vi "Main.vi"() -> ()   [LabVIEW 2017]
uses:
  Controls/MHLData.ctl
  Controls/objectRefsMain.ctl
  <vilib>/Utility/miscctls.llb/LVPositionTypeDef.ctl
  <vilib>/Utility/error.llb/DialogType.ctl
  7da0cd4f-55e9-4c1f-8356-bed5fd081df9.vi
  20102e64-79ad-4bb2-912e-c55f23ce2fb7.vi
  581ba121-4117-45c7-b05f-45eec266b530.vi
  Support/Configuration/globalConstants.vi
  <vilib>/Utility/error.llb/Error Cluster From Error Code.vi
  <vilib>/ErrorRing/Error Ring.xnode
  Support/Configuration/Message Queues/Message Queue.lvlib
  Support/Configuration/User Events/User Event - Stop.lvlib
  user32.dll
panel:
  in  "Excel._Application":refnum<k7>
  out "IL RL Standards":T1
  out "Channel Select":bool[](array[boolean])
  out "Save File":refnum<file>
  out "Device ID":refnum<visa-resource-name>="GPIB0::17::INSTR" caption="VISA resource name"
  out "experiorLogo":picture
  out "statusMessage":string="Loading Experior IL-RL"
  out "Running":bool
  in  "New Test":bool
  in  "Engineering Mode":bool
  in  "abort":bool caption="Abort"
  in  "Remeasure":bool caption="Redo"
  in  "Method Selection":u16(ring) items=["Select IL Method", "---------------------", "Standard IL", "Substitution"]
  in  "Standard Selection":u16(ring) items=["Select Test Standard", "---------------------", "No Standard", "Custom Standard", "---------------------", "GR326-UPC-New ", "GR326-UPC-During/End", "GR326-APC-New ", "GR326-APC-During/End", "GR1435-Standard-New", "GR1435-Standard-During/End"]
  in  "Rereference":bool caption="Redo"
  in  "Sample ID":string caption="Sample Number"
  in  "Enable RL":bool
  in  "Enable IL":bool
  in  "Enable Switch":bool
  in  "Wavelength Enable":T2
  in  "Channel Cluster":T3
  in  "Save Data":bool
  in  "Take Measurement":bool
  in  "Take Reference":bool
  in  "menuSlider":bool
  in  "moduleSlider":bool
  in  "Open Save":bool
  out "Save Path":string="C:\\_Labtech\\"
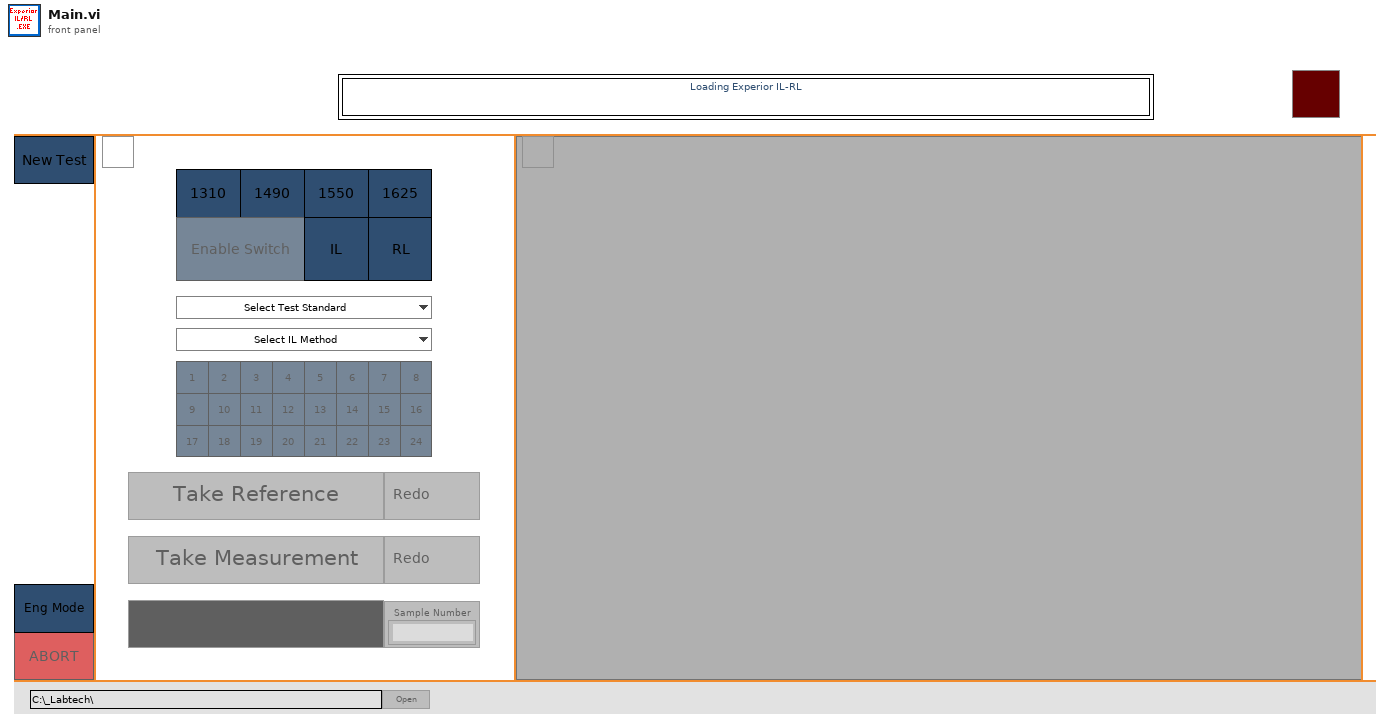
[diagram p1: front panel]
types:
  T1 = cluster{"Standard Name":string, "Max IL to Pass (dB)":dbl, "Min RL to Pass (dB)":dbl}
  T2 = cluster{"Enable RL":bool, "Enable RL 2":bool, "Enable RL 3":bool, "Enable RL 4":bool}
  T3 = cluster{"1":bool, "2":bool, "3":bool, "4":bool, "5":bool, "6":bool, "7":bool, "8":bool, "9":bool, "10":bool, "11":bool, "12":bool, "13":bool, "14":bool, "15":bool, "16":bool, "17":bool, "18":bool, "19":bool, "20":bool, "21":bool, "22":bool, "23":bool, "24":bool}
  T4 = typedef "objectRefsMain.ctl" = cluster{"experiorLogoRef":refnum<vi>, "menuSplitter1Ref":refnum<vi>, "moduleSplitter1Ref":refnum<vi>, "moduleSplitter2Ref":refnum<vi>, "statusMessageSplitterRef":refnum<vi>, "logoSplitter1Ref":refnum<vi>, "logoSplitter2Ref":refnum<vi>, "logoPaneRef":refnum<vi>, "titlePaneRef":refnum<vi>, "menuPane1Ref":refnum<vi>, "modulePane1Ref":refnum<vi>, "modulePane2Ref":refnum<vi>, "modulePane3Ref":refnum<vi>, "statusMessagePaneRef":refnum<vi>, "abortRef":refnum<vi>, "menuSliderRef":refnum<vi>, "moduleSliderRef":refnum<vi>, "statusMessageRef":refnum<vi>, "SubVISubpanelRef":refnum<vi>, "moduleSplitter3Ref":refnum<vi>, "modulePane4Ref":refnum<vi>, "deviceIdRef":refnum<vi>, "SaveFileRef":refnum<vi>, "SampleIDRef":refnum<vi>, "ChannelRef":refnum<vi>, "UseSwitchRef":refnum<vi>, "MeasButtonRef":refnum<vi>, "RefButtonRef":refnum<vi>, "SaveButtonRef":refnum<vi>, "EnlableIlRef":refnum<vi>, "EnlableRlRef":refnum<vi>, "WavelengthRef":refnum<vi>, "ChannelClusterRef":refnum<vi>, "RunTimeRef":refnum<vi>, "RereferenceRef":refnum<vi>, "RemeasureRef":refnum<vi>, "EngModeRef":refnum<vi>, "StandardSelectRef":refnum<vi>, "MethodSelectRef":refnum<vi>, "StandardRef":refnum<vi>, "SavePathRef":refnum<vi>}
  T5 = typedef "MHLData.ctl" = cluster{"objectRefsMain":T4, "SubVIExit?":bool, "statusMessage":string}
  T6 = typedef "Message Queue.lvlib/messageQueues.ctl" = cluster{"MHL":refnum<queue>, "SubVI":refnum<queue>}
  T7 = typedef "SubViRefs.ctl" = cluster{"SubViRef":refnum<vi>, "Has Switch":bool, "No Device":bool}
  T8 = typedef "notifiers.lvlib/notifiers.ctl" = cluster{"exitSubVI":refnum<notifier>}
  T9 = typedef "User Event - Stop.lvlib/userEvents.ctl" = cluster{"stop":refnum<user-event>, "sendRefs":refnum<user-event>, "sendSubVIRefs":refnum<user-event>, "eventRegRef":refnum<event-registration>}
  T10 = cluster{"queueName":string, "queueMessage":string, "priority?":bool}[]
  T11 = enum8{"Enabled", "Disabled", "Disabled and Grayed Out"}
  T12 = cluster{"IL Array":cluster{"Data Output":string, "Fail":bool}[], "RL Array":cluster{"Data Output":string, "Fail":bool}[], "Ref Power Array":string[], "Power Array":string[], "Optional Data Array":cluster{"Data Output":string, "Fail":bool}[], "Optional Param":string}
  T13 = cluster{"Enable 1310":bool, "Enable 1490":bool, "Enable 1550":bool, "Enable 1625":bool}
  T14 = typedef "DialogType.ctl" = u16
  T15 = cluster{"Value":refnum<visa-resource-name>, "Has Switch":bool}
  T16 = cluster{"Wavelength Enable":bool[], "Channel Cluster":bool[], "Enable IL":bool, "Enable RL":bool, "Enable Switch":bool, "Method Selection":u16, "Value":cluster{"Standard Name":string, "Max IL to Pass (dB)":dbl, "Min RL to Pass (dB)":dbl}}
  T17 = cluster{"Standard Name":string, "Max IL to Pass (dB)":dbl, "Min RL to Pass (dB)":dbl}[]
  T18 = typedef "LVPositionTypeDef.ctl" = cluster{"Left":i32, "Top":i32}
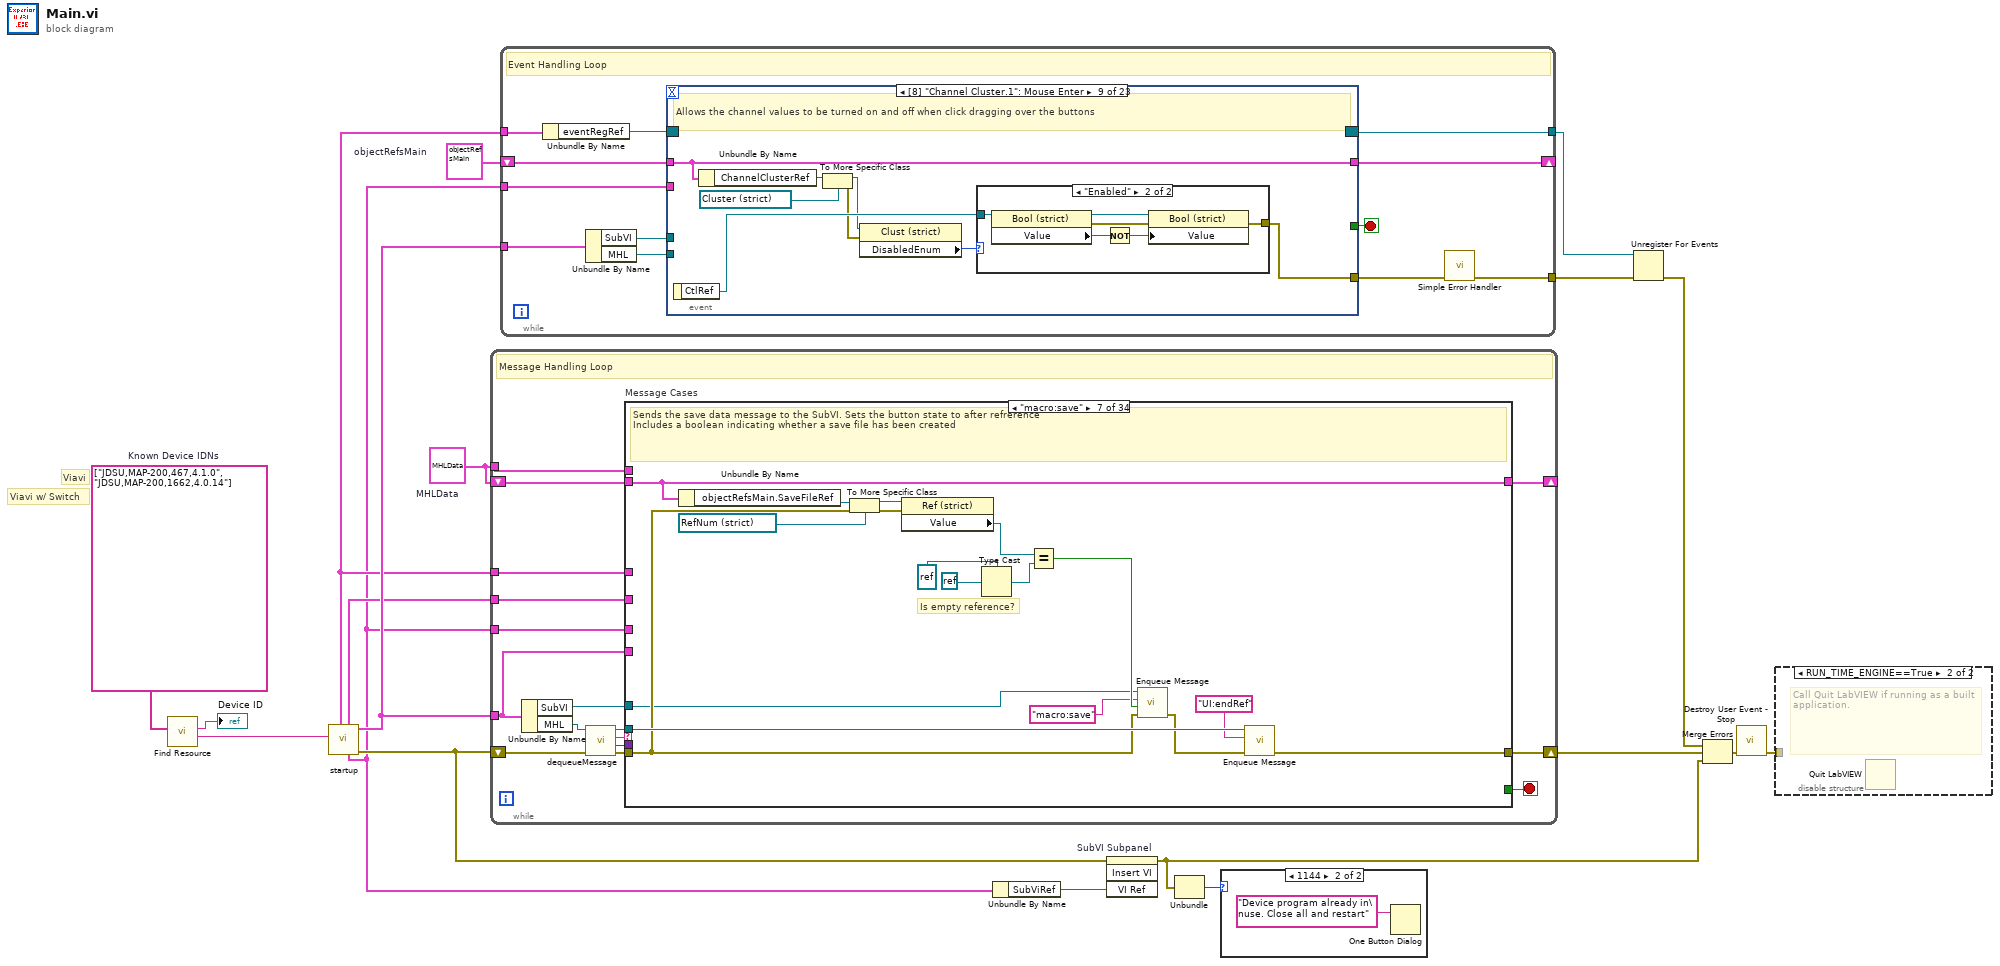
[diagram p0: block diagram]
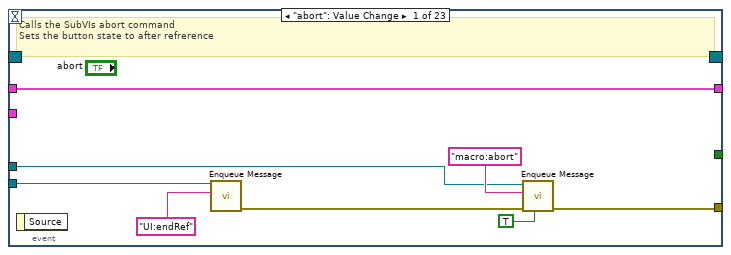
[diagram p4: hidden frame]
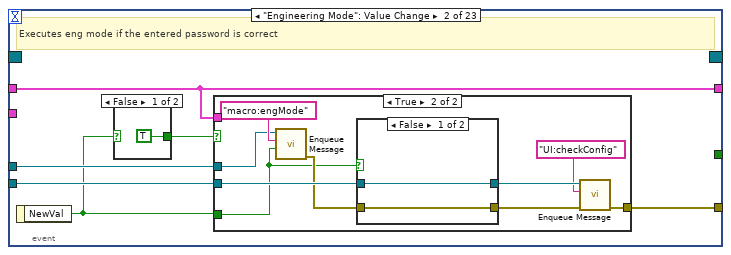
[diagram p5: hidden frame]
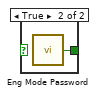
[diagram p6: hidden frame]
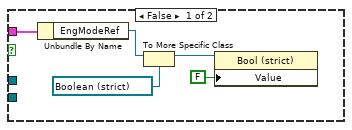
[diagram p7: hidden frame]
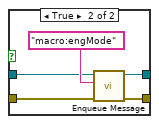
[diagram p8: hidden frame]
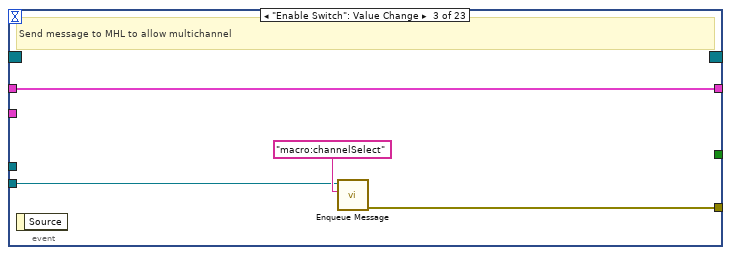
[diagram p9: hidden frame]
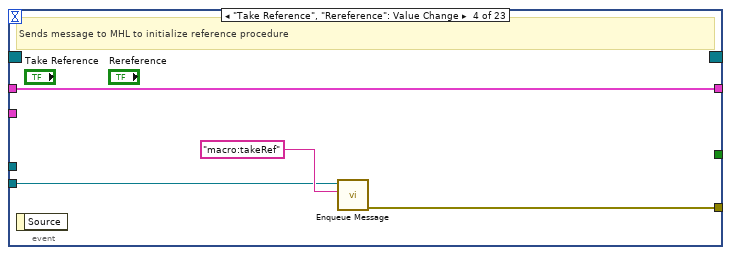
[diagram p10: hidden frame]
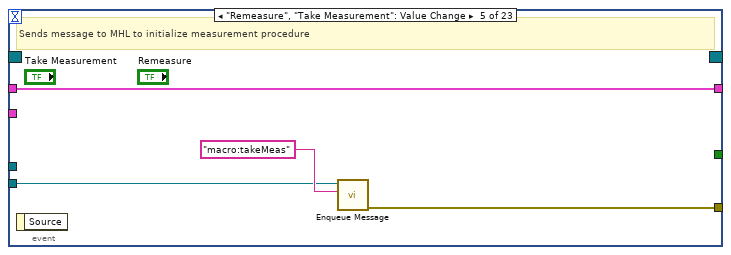
[diagram p11: hidden frame]
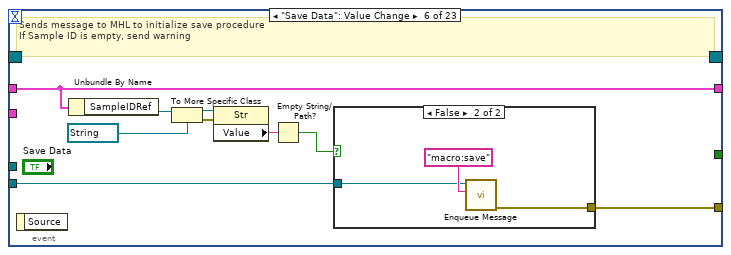
[diagram p12: hidden frame]
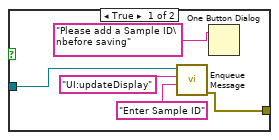
[diagram p13: hidden frame]
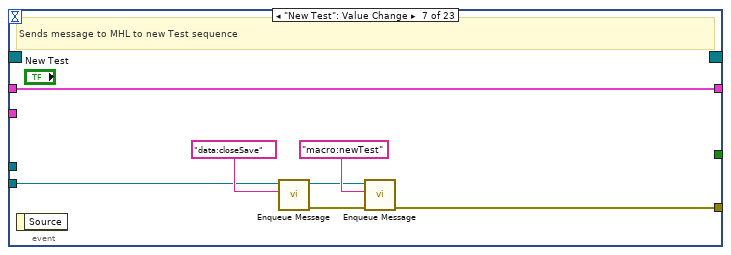
[diagram p14: hidden frame]
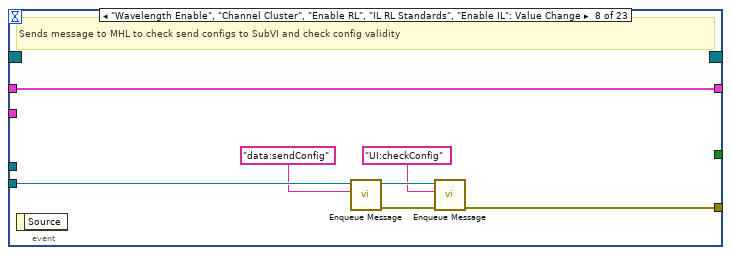
[diagram p15: hidden frame]
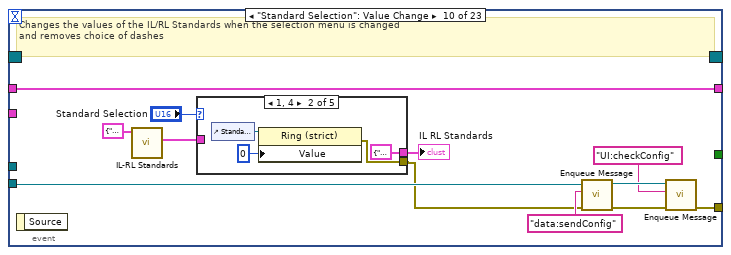
[diagram p17: hidden frame]
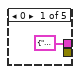
[diagram p18: hidden frame]
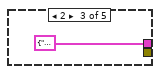
[diagram p19: hidden frame]
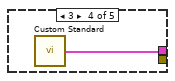
[diagram p20: hidden frame]
diagram:
  w6 = string[] ["JDSU,MAP-200,467,4.1.0", "JDSU,MAP-200,1662,4.0.14"]  # Known Device IDNs
  w9 = T4 {"experiorLogoRef"=refnum, "menuSplitter1Ref"=refnum, "moduleSplitter1Ref"=refnum, "moduleSplitter2Ref"=refnum, "statusMessageSplitterRef"=refnum, "logoSplitter1Ref"=refnum, "logoSplitter2Ref"=refnum, "logoPaneRef"=refnum, "titlePaneRef"=refnum, "menuPane1Ref"=refnum, "modulePane1Ref"=refnum, "modulePane2Ref"=refnum, "modulePane3Ref"=refnum, "statusMessagePaneRef"=refnum, "abortRef"=refnum, "menuSliderRef"=refnum, "moduleSliderRef"=refnum, "statusMessageRef"=refnum, "SubVISubpanelRef"=refnum, "moduleSplitter3Ref"=refnum, "modulePane4Ref"=refnum, "deviceIdRef"=refnum, "SaveFileRef"=refnum, "SampleIDRef"=refnum, "ChannelRef"=refnum, "UseSwitchRef"=refnum, "MeasButtonRef"=refnum, "RefButtonRef"=refnum, "SaveButtonRef"=refnum, "EnlableIlRef"=refnum, "EnlableRlRef"=refnum, "WavelengthRef"=refnum, "ChannelClusterRef"=refnum, "RunTimeRef"=refnum, "RereferenceRef"=refnum, "RemeasureRef"=refnum, "EngModeRef"=refnum, "StandardSelectRef"=refnum, "MethodSelectRef"=refnum, "StandardRef"=refnum, "SavePathRef"=refnum}  # objectRefsMain
  w12 = T5 {"objectRefsMain"={"experiorLogoRef"=refnum, "menuSplitter1Ref"=refnum, "moduleSplitter1Ref"=refnum, "moduleSplitter2Ref"=refnum, "statusMessageSplitterRef"=refnum, "logoSplitter1Ref"=refnum, "logoSplitter2Ref"=refnum, "logoPaneRef"=refnum, "titlePaneRef"=refnum, "menuPane1Ref"=refnum, "modulePane1Ref"=refnum, "modulePane2Ref"=refnum, "modulePane3Ref"=refnum, "statusMessagePaneRef"=refnum, "abortRef"=refnum, "menuSliderRef"=refnum, "moduleSliderRef"=refnum, "statusMessageRef"=refnum, "SubVISubpanelRef"=refnum, "moduleSplitter3Ref"=refnum, "modulePane4Ref"=refnum, "deviceIdRef"=refnum, "SaveFileRef"=refnum, "SampleIDRef"=refnum, "ChannelRef"=refnum, "UseSwitchRef"=refnum, "MeasButtonRef"=refnum, "RefButtonRef"=refnum, "SaveButtonRef"=refnum, "EnlableIlRef"=refnum, "EnlableRlRef"=refnum, "WavelengthRef"=refnum, "ChannelClusterRef"=refnum, "RunTimeRef"=refnum, "RereferenceRef"=refnum, "RemeasureRef"=refnum, "EngModeRef"=refnum, "StandardSelectRef"=refnum, "MethodSelectRef"=refnum, "StandardRef"=refnum, "SavePathRef"=refnum}, "SubVIExit?"=FALSE, "statusMessage"=""}  # MHLData
  # "Viavi w/ Switch"
  # "Viavi"
  n1 = call "Find Resource.vi"("Known Device IDN"=w6) -> ("Return IDN"=w4:string, "Resource Name"=→"Device ID":string)  [unwired: 8 in, 1 out]
  n2 = call "startup.vi"("Device IDN"=w4) -> ("error out"=w8:errorcluster, "messageQueues"=w14:T6, "SubViRefs"=w3:T7, "Notifiers"=w13:T8, "userEvents"=w10:T9)  [unwired: 6 in]
  n3 = while {
    tunnel: w14 -> [w23]
    shift-right: [w31] -> w15
    shift-left: w8 -> [w34]
    tunnel: w13 -> [w30]
    tunnel: w3 -> [w27]
    shift-right: [w25] -> _
    shift-left: w12 -> [w26]
    tunnel: w12 -> [w24]
    tunnel: w10 -> [w22]
    stop <- w35 stop-if-true
    # "Message Handling Loop"
    n4 = Unbundle By Name(w23) -> ("SubVI"=w20:refnum<queue>, "MHL"=w29:refnum<queue>)
    n5 = call "dequeueMessage.vi"("error in (no error)"=w34, "Message Queue"=w29) -> ("error out"=w21:errorcluster, "Message Data"=w32:variant, "Message"=w33:string, "dup Message Queue"=w28:refnum<queue>)  [unwired: 6 in]
    n6 = case "Message Cases" shown="\"macro:save\"" w33 {
      selector: w33 -> [_ _ _ _ _ _ _ _ _ _ _ w165 _ _ _ _ _ _ _ _ _ _ _ _ _ _ _ _ _ _ _ _ _ _]
      tunnel: w28 -> [_ _ w45 _ _ _ w118 _ _ w156 _ _ _ w212 w251 _ _ _ _ _ _ _ _ _ w404 w461 _ _ w579 w621 _ _ _ _]
      tunnel: w21 -> [w37 w41 w46 w81 w100 w105 w117 w134 w150 w155 w164 _ w194 w208 w252 w255 w256 w268 w278 w314 w320 w367 w377 w380 w406 w449 w499 w537 w576 w618 w660 w711 w723 w736]
      tunnel: [w37 w40 w43 w81 w103 w108 w110 w135 w151 w160 w164 w166 w176 w219 w248 w255 w260 w272 w292 w308 w328 w371 w377 w378 w405 w464 w499 w537 w578 w620 w660 w711 w723 w728] -> w31
      tunnel: w26 -> [w36 w42 w49 w80 w104 w109 w115 w127 w153 w162 w163 w167 w193 w217 w253 w254 w263 w267 w283 w319 w322 w366 w376 w379 w383 w442 w500 w539 w581 w623 w661 w702 w714 w733]
      tunnel: [w36 w42 w49 w80 w104 w109 w115 w127 w153 w162 w163 w167 w193 w220 w253 w254 w264 w267 w283 w319 w322 w366 w376 w379 w383 w442 w500 w539 w581 w623 w661 w702 w714 w731] -> w25
      tunnel: [_ _ _ _ _ _ _ _ _ _ _ _ _ _ TRUE _ _ _ _ _ _ _ _ _ _ _ _ _ _ _ _ _ _ _] -> w35
      tunnel: w32 -> [_ _ _ _ _ _ _ _ _ _ _ _ w192 w209 _ _ _ _ _ w313 w350 _ _ _ _ _ _ _ _ _ _ _ _ w734]
      tunnel: w20 -> [_ _ _ _ _ _ w111 _ w149 _ _ _ _ _ _ _ _ w269 w290 w307 _ _ _ _ _ _ _ _ _ _ _ _ _ _]
      tunnel: w30 -> [_ _ _ _ _ _ _ _ _ _ _ _ _ w218 _ _ _ _ _ _ _ _ _ _ _ _ _ _ _ _ _ _ _ _]
      tunnel: w27 -> [_ _ _ w89 _ _ _ _ _ _ _ _ _ w207 _ _ _ w266 _ _ _ _ _ _ _ _ _ _ _ _ w688 _ _ _]
      tunnel: w24 -> [_ _ _ _ _ _ _ _ _ _ _ _ _ _ _ _ _ _ _ _ _ _ _ _ _ _ _ _ _ _ _ _ _ _]
      tunnel: w23 -> [_ w39 _ _ w102 w107 _ w133 w148 w157 _ _ _ _ _ _ _ _ _ _ _ _ _ _ _ _ _ _ _ _ _ _ _ _]
      tunnel: w22 -> [_ _ _ _ _ _ _ _ _ _ _ _ _ _ w247 _ w258 _ _ _ _ _ _ _ _ _ _ _ _ _ _ _ _ _]
      frame "---------- Macro ----------" {
        # "Template Separator\n(You can make a copy of, or modify, this frame)"
      }
      frame "macro:init" {
        # "This case sends sequential queue message(s). Do not execute any code in this case.\nStartup procedure."
        n7 = call "sendMultipleMessages.vi"("error in (no error)"=w41, "queueMessages"=T10 [{"queueName"="MHL", "queueMessage"="data:init", "priority?"=FALSE}, {"queueName"="MHL", "queueMessage"="UI:init", "priority?"=FALSE}, {"queueName"="MHL", "queueMessage"="data:sendInit", "priority?"=FALSE}, {"queueName"="MHL", "queueMessage"="macro:newTest", "priority?"=FALSE}, {"queueName"="MHL", "queueMessage"="UI:endRun", "priority?"=FALSE}], "messageQueues"=w39) -> ("error out"=w40:errorcluster)  [unwired: 8 in]
      }
      frame "macro:engMode" {
        # "Sets all buttons and configs to enabled"
        n8 = call "Enqueue Message.vi"("error in (no error)"=w46, "Message"="UI:enableConfig", "Message Queue"=w45) -> ("error out"=w43:errorcluster)  [unwired: 7 in, 1 out]
        n9 = Unbundle By Name(w49) -> ("objectRefsMain.RefButtonRef"=w55:refnum<vi>, "objectRefsMain.RereferenceRef"=w54:refnum<vi>, "objectRefsMain.MeasButtonRef"=w53:refnum<vi>, "objectRefsMain.RemeasureRef"=w52:refnum<vi>, "objectRefsMain.SaveButtonRef"=w51:refnum<vi>, "objectRefsMain.SampleIDRef"=w50:refnum<vi>)
        n10 = To More Specific Class(target class=refnum<vi> refnum ("Save Data"), reference=w55, error in=w43) -> (specific class reference=w75:refnum<vi>, error out=w77:errorcluster)
        n11 = To More Specific Class(target class=refnum<vi> refnum ("Save Data"), reference=w54, error in=w43) -> (specific class reference=w70:refnum<vi>, error out=w73:errorcluster)
        n12 = To More Specific Class(target class=refnum<vi> refnum ("Save Data"), reference=w53, error in=w43) -> (specific class reference=w67:refnum<vi>, error out=w69:errorcluster)
        n13 = To More Specific Class(target class=refnum<vi> refnum ("Save Data"), reference=w52, error in=w43) -> (specific class reference=w62:refnum<vi>, error out=w65:errorcluster)
        n14 = To More Specific Class(target class=refnum<vi> refnum ("Save Data"), reference=w51, error in=w43) -> (specific class reference=w58:refnum<vi>, error out=w61:errorcluster)
        n15 = To More Specific Class(target class=refnum<vi> refnum ("Sample ID"), reference=w50, error in=w43) -> (specific class reference=w56:refnum<vi>, error out=w57:errorcluster)
        n16 = property class="Bool"(reference=w75, error in=w77, "DisabledEnum"=T11."Enabled" ("Disabled")) -> ()  [unwired: 2 out]
        n17 = property class="Bool"(reference=w70, error in=w73, "DisabledEnum"=T11."Enabled" ("Disabled")) -> ()  [unwired: 2 out]
        n18 = property class="Bool"(reference=w67, error in=w69, "DisabledEnum"=T11."Enabled" ("Disabled")) -> ()  [unwired: 2 out]
        n19 = property class="Bool"(reference=w62, error in=w65, "DisabledEnum"=T11."Enabled" ("Disabled")) -> ()  [unwired: 2 out]
        n20 = property class="Bool"(reference=w58, error in=w61, "DisabledEnum"=T11."Enabled" ("Disabled")) -> ()  [unwired: 2 out]
        n21 = property class="Str"(reference=w56, error in=w57, "DisabledEnum"=T11."Enabled" ("Disabled")) -> ()  [unwired: 2 out]
      }
      frame "macro:channelSelect" {
        # "Forces \"Use Switch\" off when device has no switch"
        # "Enables or disables multichannel functionality\nCompletely disables multichannel when no switch detected"
        n22 = Unbundle By Name(w80) -> ("objectRefsMain.ChannelClusterRef"=w83:refnum<vi>)
        n23 = Unbundle By Name(w80) -> ("objectRefsMain.UseSwitchRef"=w88:refnum<vi>)
        n24 = Unbundle By Name(w89) -> ("Has Switch"=w78:bool)
        n25 = To More Specific Class(target class=refnum<vi> refnum ("Channel Cluster"), reference=w83, error in=w81) -> (specific class reference=w82:refnum<vi>)  [unwired: 1 out]
        n26 = To More Specific Class(target class=refnum<vi> refnum ("Single Channel"), reference=w88, error in=w81) -> (specific class reference=w84:refnum<vi>, error out=w86:errorcluster)
        n27 = property class="Bool (strict)"(reference=w84, error in=w86) -> ("Value"=w85:bool)  [unwired: 2 out]
        n28 = case shown="True" w78 {
          tunnel: w84 -> [w95 w99]
          tunnel: w81 -> [w93 w98]
          frame True {
            n29 = property class="Bool (strict)"(reference=w95, error in=w93, "DisabledEnum"=T11."Enabled" ("Disabled")) -> ()  [unwired: 2 out]
          }
          frame False {
            n30 = property class="Bool (strict)"(reference=w99, error in=w98, "Value"=FALSE, "DisabledEnum"=T11."Disabled and Grayed Out" ("Disabled")) -> ()  [unwired: 2 out]
          }
        }
        n31 = Select(t=0, s=w85, f=2) -> (s? t:f=w92:i32)
        n32 = property class="Clust (strict)"(reference=w82, "DisabledEnum"=w92) -> ()  [unwired: 1 in, 2 out]
      }
      frame "macro:takeRef" {
        # "Calls the SubVIs takeRef command\nDisables configs, temporarily disables buttons"
        n33 = call "sendMultipleMessages.vi"("error in (no error)"=w100, "queueMessages"=T10 [{"queueName"="SubVI", "queueMessage"="macro:takeRef", "priority?"=FALSE}, {"queueName"="MHL", "queueMessage"="UI:disableButton", "priority?"=FALSE}, {"queueName"="MHL", "queueMessage"="UI:disableConfig", "priority?"=FALSE}], "messageQueues"=w102) -> ("error out"=w103:errorcluster)  [unwired: 8 in]
      }
      frame "macro:takeMeas" {
        # "Calls the SubVIs takeMeas command\nDisables configs, temporarily disables buttons"
        n34 = call "sendMultipleMessages.vi"("error in (no error)"=w105, "queueMessages"=T10 [{"queueName"="SubVI", "queueMessage"="macro:takeMeas", "priority?"=FALSE}, {"queueName"="MHL", "queueMessage"="UI:disableButton", "priority?"=FALSE}, {"queueName"="MHL", "queueMessage"="UI:disableConfig", "priority?"=FALSE}], "messageQueues"=w107) -> ("error out"=w108:errorcluster)  [unwired: 8 in]
      }
      frame "macro:save" {
        # "Is empty reference?"
        # "Sends the save data message to the SubVI. Sets the button state to after refrerence\nIncludes a boolean indicating whether a save file has been created"
        n35 = Unbundle By Name(w115) -> ("objectRefsMain.SaveFileRef"=w125:refnum<vi>)
        n36 = To More Specific Class(target class=refnum<vi> refnum ("refnum"), reference=w125, error in=w117) -> (specific class reference=w119:refnum<vi>, error out=w126:errorcluster)
        n37 = property class="Ref (strict)"(reference=w119, error in=w126) -> ("Value"=w123:refnum<file>)  [unwired: 2 out]
        n38 = Type Cast(type=refnum<file> refnum ("Byte Stream File Refnum"), x=refnum<k0> refnum) -> (*(type *) &x=w120:refnum<file>)
        n39 = Equal?(x=w123, y=w120) -> (x = y?=w116:bool)
        n40 = call "Enqueue Message.vi"("error in (no error)"=w117, "Message Data"=w116, "Message"="macro:save", "Message Queue"=w111) -> ("error out"=w112:errorcluster)  [unwired: 6 in, 1 out]
        n41 = call "Enqueue Message.vi"("error in (no error)"=w112, "Message"="UI:endRef", "Message Queue"=w118) -> ("error out"=w110:errorcluster)  [unwired: 7 in, 1 out]
      }
      frame "macro:newTest" {
        # "Sets save file to null value"
        # "Reinitializes values, buttons, configs, and removes \nCalls the SubVIs newTest command"
        n42 = Unbundle By Name(w127) -> ("objectRefsMain.SaveFileRef"=w140:refnum<vi>)
        n43 = Unbundle By Name(w127) -> ("objectRefsMain.SavePathRef"=w130:refnum<vi>)
        n44 = To More Specific Class(target class=refnum<vi> refnum ("Save Path"), reference=w130) -> (specific class reference=w128:refnum<vi>)  [unwired: 1 in, 1 out]
        n45 = To More Specific Class(target class=refnum<vi> refnum ("refnum"), reference=w140, error in=w134) -> (specific class reference=w141:refnum<vi>, error out=w142:errorcluster)
        n46 = Type Cast(type=refnum<file> refnum ("Byte Stream File Refnum"), x=refnum<k0> refnum) -> (*(type *) &x=w136:refnum<file>)
        n47 = property class="Str"(reference=w128, "Value"="C:\\_Labtech\\") -> ()  [unwired: 1 in, 2 out]
        n48 = property class="Ref (strict)"(reference=w141, error in=w142, "Value"=w136) -> ()  [unwired: 2 out]
        n49 = call "sendMultipleMessages.vi"("error in (no error)"=w134, "queueMessages"=T10 [{"queueName"="MHL", "queueMessage"="UI:initConfig", "priority?"=FALSE}, {"queueName"="MHL", "queueMessage"="UI:checkConfig", "priority?"=FALSE}, {"queueName"="MHL", "queueMessage"="UI:enableConfig", "priority?"=FALSE}, {"queueName"="MHL", "queueMessage"="macro:channelSelect", "priority?"=FALSE}, {"queueName"="SubVI", "queueMessage"="macro:newTest", "priority?"=FALSE}], "messageQueues"=w133) -> ("error out"=w135:errorcluster)  [unwired: 8 in]
      }
      frame "macro:initExit" {
        # "Waits for SubVi to abort current Queue\nbefore sending exit command"
        # "Initiates shutdown procedure. Subpanel processes exit, MHL exit, EHL exit.\nSafely aborts all messages within the SubVI then initializes exit"
        n50 = call "Enqueue Message.vi"("Priority Message? (F)"=TRUE, "error in (no error)"=w150, "Message"="macro:abort", "Message Queue"=w149) -> ("error out"=w145:errorcluster)  [unwired: 6 in, 1 out]
        n51 = call "Stall Data Flow.vim"("value in"=w145, "milliseconds to wait"=500) -> ("value out"=w144:errorcluster)  [unwired: 1 out]
        n52 = call "sendMultipleMessages.vi"("error in (no error)"=w144, "queueMessages"=T10 [{"queueName"="MHL", "queueMessage"="core:waitOnSubVIExit", "priority?"=FALSE}, {"queueName"="SubVI", "queueMessage"="macro:exit", "priority?"=FALSE}], "messageQueues"=w148) -> ("error out"=w151:errorcluster)  [unwired: 8 in]
      }
      frame "macro:exit" {
        # "Shutdown procedure."
        n53 = call "Enqueue Message.vi"("error in (no error)"=w155, "Message Data"="Closing program.", "Message"="UI:updateDisplay", "Message Queue"=w156) -> ("error out"=w154:errorcluster)  [unwired: 6 in, 1 out]
        n54 = call "sendMultipleMessages.vi"("error in (no error)"=w154, "queueMessages"=T10 [{"queueName"="MHL", "queueMessage"="UI:init", "priority?"=FALSE}, {"queueName"="MHL", "queueMessage"="data:init", "priority?"=FALSE}, {"queueName"="MHL", "queueMessage"="data:closeSave", "priority?"=FALSE}, {"queueName"="MHL", "queueMessage"="core:exit", "priority?"=FALSE}], "messageQueues"=w157) -> ("error out"=w160:errorcluster)  [unwired: 8 in]
      }
      frame "---------- Core ----------" {
        # "Template Separator\n(You can make a copy of, or modify, this frame)"
      }
      frame Default {
        # "'Default' case only runs if there is a message that isn't defined in any of the other cases.  Output a programming error."
        n55 = xnode "Error Ring"("parameter 0"=w165) -> ("error out"=w166:errorcluster)
      }
      frame "core:error" {
        w182 = T14 0 items=["no dialog", "OK message", "continue or stop message", "OK message + warnings", "continue/stop + warnings"]  # type of dialog (OK msg:1)
        # "Add case for user made error message"
        # "Open Error Log.txt, Log error, close file, notify user, clear errors."
        n56 = Variant To Data(error in=w194, type=errorcluster {"status"=FALSE, "code"=0, "source"=""} ("error constant"), Variant=w192) -> (data=w189:errorcluster, error out=w190:errorcluster)
        n57 = Merge Errors(w189, w190) -> (w188:errorcluster)
        n58 = Unbundle By Name(w188) -> ("code"=w175:i32, "source"=w178:string)
        n59 = call <vilib>:"General Error Handler.vi"("[error code] (0)"=w175, "[error source] (\" \")"=w178, "type of dialog (OK msg:1)"=w182) -> ("code out"=w183:i32, "message"=w177:string)  [unwired: 8 in, 3 out]
        n60 = call "CreateErrorLog.vi"() -> ("error out"=w181:errorcluster, "refnum out"=w180:refnum<file>)  [unwired: 10 in]
        n61 = call "Log Error.vi"("Error Message"=w177, "error in"=w181, "Source"=w178, "Code"=w183, "Error Log Refnum In"=w180) -> ("error out"=w186:errorcluster, "Error Log Refnum Out"=w185:refnum<file>)  [unwired: 5 in]
        n62 = Not A Number/Path/Refnum?(number/path/refnum=w185) -> (NaN/Path/Refnum?=w187:bool)
        n63 = case "EmptyPath?" shown="False" w187 {
          tunnel: [w203 w204] -> w184
          tunnel: w186 -> [w202 w204]
          tunnel: w185 -> [w201 _]
          frame False {
            n64 = Close File(refnum=w201, error in=w202) -> (error out=w203:errorcluster)  [unwired: 1 out]
          }
          frame True {
          }
        }
        n65 = case shown="1000" w175 {
          tunnel: w184 -> [w198 w200]
          tunnel: w175 -> [w197 _]
          tunnel: [w196 w200] -> w179
          tunnel: w178 -> [w195 _]
          frame 0, Default {
            n66 = call <vilib>:"General Error Handler.vi"("[error code] (0)"=w197, "[error source] (\" \")"=w195, "error in (no error)"=w198) -> ("error out"=w196:errorcluster)  [unwired: 8 in, 4 out]
          }
          frame 1000 {
            # "Error 1000:\nCannot initialize SubVI"
            n67 = One Button Dialog(message="Could not connect to device\nExiting out of program") -> ()  [unwired: 1 in, 1 out]
          }
        }
        n68 = call <vilib>:"Clear Errors.vi"("error in (no error)"=w179) -> ("error out"=w176:errorcluster)  [unwired: 5 in, 1 out]
      }
      frame "core:waitOnSubVIExit" {
        # "If no SubVI initialized,\nskip exit proceedure"
        # "Keep checking for exit notification until received. When TML,TCL, and CCL Exit notifications recieved, exit MHL"
        n69 = Unbundle By Name(w207) -> ("No Device"=w205:bool)
        n70 = Unbundle By Name(w217) -> ("SubVIExit?"=w215:bool)
        n71 = Unbundle By Name(w218) -> ("exitSubVI"=w214:refnum<notifier>)
        n72 = case shown="False" w205 {
          tunnel: w214 -> [_ w236]
          tunnel: [TRUE ("processExit?") w235] -> w213
          tunnel: w212 -> [w223 w234]
          tunnel: [w221 w233] -> w211
          tunnel: [w223 w232] -> w210
          tunnel: w209 -> [_ w230]
          tunnel: w208 -> [w221 w228]
          frame True {
          }
          frame False {
            # "Handles first exit call"
            n73 = Variant To Data(error in=w228, type=0, Variant=w230) -> (data=w227:i32, error out=w225:errorcluster)
            n74 = case shown="Error" w225 {
              selector: w225 -> [w237 _]
              tunnel: w227 -> [w239 _]
              tunnel: [w238 0] -> w226
              tunnel: [w237 _] -> w224
              frame No Error {
                n75 = Increment(x=w239) -> (x+1=w238:i32)
              }
              frame Error {
              }
            }
            n76 = call "waitOnProcessExit.vi"("Timeout Exit"=w226, "error in (no error)"=w224, "Message"="core:waitOnSubVIExit", "MHL"=w234, "notifier"=w236) -> ("error out"=w233:errorcluster, "MHLDup"=w232:refnum<queue>, "processExit?"=w235:bool)  [unwired: 4 in]
          }
        }
        n77 = Select(t=w213, s=w213, f=w215) -> (s? t:f=w216:bool)
        n78 = Bundle By Name(cluster=w217, "SubVIExit?"=w216) -> (w220:T5)
        n79 = Unbundle By Name(w220) -> ("SubVIExit?"=w206:bool)
        n80 = case "ExitMHL?" shown="True" w206 {
          tunnel: [w241 w245] -> w219
          tunnel: w210 -> [_ w244]
          tunnel: w211 -> [w241 w243]
          frame False {
          }
          frame True {
            n81 = call "Enqueue Message.vi"("error in (no error)"=w243, "Message"="macro:exit", "Message Queue"=w244) -> ("error out"=w245:errorcluster)  [unwired: 7 in, 1 out]
          }
        }
      }
      frame "core:exit" {
        # "Release MHLQueue, Fire User Stop Event to Exit EHL, Exit MHL"
        n82 = Release Queue(queue=w251, error in (no error)=w252) -> (error out=w250:errorcluster)  [unwired: 1 in, 2 out]
        n83 = Unbundle By Name(w247) -> ("stop"=w246:refnum<user-event>)
        n84 = call "fireEventStop.vi"("error in (no error)"=w250, "stop"=w246) -> ("error out"=w248:errorcluster)  [unwired: 9 in]
      }
      frame "---------- Data ----------" {
        # "Template Separator\n(You can make a copy of, or modify, this frame)"
      }
      frame "data:init" {
        # "Open object references."
        n85 = Unbundle By Name(w258) -> ("sendRefs"=w257:refnum<user-event>)
        n86 = Unbundle By Name(w263) -> ("objectRefsMain"=w262:T4)
        n87 = call "openRefsMain.vi"("error in (no error)"=w256, "objectRefsMain"=w262) -> ("error out"=w261:errorcluster, "objectRefsMainOut"=w259:T4)  [unwired: 6 in, 2 out]
        n88 = Bundle By Name(cluster=w263, "objectRefsMain"=w259) -> (w264:T5)
        n89 = call "fireEventSendRefs.vi"("error in (no error)"=w261, "objectRefsMain"=w259, "sendRefs"=w257) -> ("error out"=w260:errorcluster)  [unwired: 8 in]
      }
      frame "data:sendInit" {
        # "Initializes variables for the sub VI\nSends variables in message data"
        n90 = Unbundle By Name(w267) -> ("objectRefsMain.deviceIdRef"=w274:refnum<vi>)
        n91 = To More Specific Class(target class=refnum<vi> refnum ("VISA resource name"), reference=w274, error in=w268) -> (specific class reference=w275:refnum<vi>, error out=w276:errorcluster)
        n92 = property class="VISAName"(reference=w275, error in=w276) -> ("Value"=w271:refnum<visa-resource-name>)  [unwired: 2 out]
        n93 = Unbundle By Name(w266) -> ("Has Switch"=w265:bool)
        n94 = Bundle("Value"=w271, "Has Switch"=w265) -> (w270:T15)  [unwired: 1 in]
        n95 = call "Enqueue Message.vi"("error in (no error)"=w268, "Message Data"=w270, "Message"="data:getInit", "Message Queue"=w269) -> ("error out"=w272:errorcluster)  [unwired: 6 in, 1 out]
      }
      frame "data:sendConfig" {
        # "Sends configs to SubVI to save\nSends variables in message data"
        n96 = Unbundle By Name(w283) -> ("objectRefsMain.StandardRef"=w282:refnum<vi>)
        n97 = To More Specific Class(target class=refnum<vi> refnum ("IL RL Standards"), reference=w282, error in=w278) -> (specific class reference=w279:refnum<vi>, error out=w280:errorcluster)
        n98 = property class="Clust (strict)"(reference=w279, error in=w280) -> ("Value"=w285:T1)  [unwired: 2 out]
        n99 = case shown="True" "Enable Switch" {
          tunnel: [bool[] [TRUE] w297] -> w289
          frame False {
          }
          frame True {
            n100 = Cluster To Array(cluster="Channel Cluster") -> (array=w297:bool[])
          }
        }
        "Channel Select" <- w289
        n101 = Cluster To Array(cluster="Wavelength Enable") -> (array=w291:bool[])
        n102 = Bundle("Wavelength Enable"=w291, "Channel Cluster"=w289, "Enable IL"="Enable IL", "Enable RL"="Enable RL", "Enable Switch"="Enable Switch", "Method Selection"="Method Selection", "Value"=w285) -> (w293:T16)  [unwired: 1 in]
        n103 = call "Enqueue Message.vi"("error in (no error)"=w278, "Message Data"=w293, "Message"="data:getConfig", "Message Queue"=w290) -> ("error out"=w292:errorcluster)  [unwired: 6 in, 1 out]
      }
      frame "data:buildSave" {
        # "Runs the VI to create a new save and its headers\nRequires a 2d string used for additional save information (leave empty if you no extra save data needed)\nRe-calls the SubVI save command"
        n104 = Variant To Data(error in=w314, type=string[][] [] ("Optional Save"), Variant=w313) -> (data=w304:string[][], error out=w312:errorcluster)
        n105 = call "Build Header.vi"("error in (no error)"=w312) -> ("error out"=w316:errorcluster, "File Path Out"=→"Save Path":string, "Header"=w299:string, "File Ref Out"=w300:refnum<file>)  [unwired: 7 in]
        n106 = Write to Text File(file (use dialog)=w300, text=w299, error in=w316) -> (refnum out=w317:refnum<file>, error out=w318:errorcluster)  [unwired: 1 in, 1 out]
        n107 = call "Column Names.vi"("Optional Save"=w304) -> ("Output"=w306:string)  [unwired: 10 in]
        n108 = Write to Text File(file (use dialog)=w317, text=w306, error in=w318) -> (refnum out=→"Save File":refnum<file>, error out=w309:errorcluster)  [unwired: 1 in, 1 out]
        n109 = control-ref of="Open Save"() -> (w303:refnum<vi>)
        n110 = property class="Bool"(reference=w303, "DisabledEnum"=T11."Enabled" ("Disabled")) -> ()  [unwired: 1 in, 2 out]
        n111 = call "Enqueue Message.vi"("error in (no error)"=w309, "Message Data"=FALSE, "Message"="macro:save", "Message Queue"=w307) -> ("error out"=w308:errorcluster)  [unwired: 6 in, 1 out]
      }
      frame "data:saveData" {
        # "Recieves temp data from the SubVI to save\nRequires a cluster arrays 2 array clusters of string and boolean, 2 string array,\nan optional extra array cluster of string and boolean, as well as a parameter for the extra array"
        n112 = Unbundle By Name(w322) -> ("objectRefsMain.SaveFileRef"=w347:refnum<vi>)
        n113 = Unbundle By Name(w322) -> ("objectRefsMain.ChannelRef"=w341:refnum<vi>)
        n114 = Unbundle By Name(w322) -> ("objectRefsMain.StandardRef"=w326:refnum<vi>)
        n115 = Unbundle By Name(w322) -> ("objectRefsMain.SampleIDRef"=w340:refnum<vi>)
        n116 = Variant To Data(error in=w320, type=T12 {"IL Array"=[], "RL Array"=[], "Ref Power Array"=[], "Power Array"=[], "Optional Data Array"=[], "Optional Param"=""} ("cluster"), Variant=w350) -> (data=w337:T12, error out=w345:errorcluster)
        n117 = To More Specific Class(target class=refnum<vi> refnum ("IL RL Standards"), reference=w326, error in=w320) -> (specific class reference=w323:refnum<vi>, error out=w324:errorcluster)
        n118 = To More Specific Class(target class=refnum<vi> refnum ("refnum"), reference=w347, error in=w320) -> (specific class reference=w348:refnum<vi>, error out=w349:errorcluster)
        n119 = To More Specific Class(target class=refnum<vi> refnum ("array"), reference=w341, error in=w320) -> (specific class reference=w342:refnum<vi>, error out=w343:errorcluster)
        n120 = To More Specific Class(target class=refnum<vi> refnum ("Sample Number"), reference=w340, error in=w320) -> (specific class reference=w336:refnum<vi>)  [unwired: 1 out]
        n121 = property class="Clust (strict)"(reference=w323, error in=w324) -> ("Value"=w321:T1)  [unwired: 2 out]
        n122 = property class="Ref (strict)"(reference=w348, error in=w349) -> ("Value"=w344:refnum<file>)  [unwired: 2 out]
        n123 = property class="Arr (strict)"(reference=w342, error in=w343) -> ("Value"=w338:bool[])  [unwired: 2 out]
        n124 = Array Size(array=w338) -> (size(s)=w332:i32)
        n125 = for {
          N: w332 -> [_]
          tunnel: w338 -> [w355] mode=indexing
          shift-right: [w352] -> w330
          shift-left: i32[] [] -> [w351]
          i -> [w354]
          n126 = Increment(x=w354) -> (x+1=w353:i32)
          n127 = case shown="True" w355 {
            tunnel: w353 -> [_ w359]
            tunnel: [w356 w358] -> w352
            tunnel: w351 -> [w356 w357]
            frame False {
            }
            frame True {
              # "Gets all enabled channels"
              n128 = Build Array (concatenate)(w357, w359) -> (w358:i32[])
            }
          }
        }
        n129 = call "Save Data.vi"("Sample ID"="Sample ID", "Channels"=w330, "Standard Input"=w321, "Input Data Arrays"=w337) -> ("Output"=w333:string)  [unwired: 7 in]
        n130 = Write to Text File(file (use dialog)=w344, text=w333, error in=w345) -> (error out=w328:errorcluster)  [unwired: 1 in, 2 out]
        n131 = property class="Str"(reference=w336, error in=w328, "Value"="") -> ()  [unwired: 2 out]
      }
      frame "data:closeSave" {
        # "Closes the current reference to the save file"
        n132 = Unbundle By Name(w366) -> ("objectRefsMain.SaveFileRef"=w368:refnum<vi>)
        n133 = To More Specific Class(target class=refnum<vi> refnum ("refnum"), reference=w368, error in=w367) -> (specific class reference=w369:refnum<vi>, error out=w370:errorcluster)
        n134 = property class="Ref (strict)"(reference=w369, error in=w370) -> ("Value"=w361:refnum<file>)  [unwired: 2 out]
        n135 = Type Cast(type=refnum<file> refnum ("Byte Stream File Refnum"), x=refnum<k0> refnum) -> (*(type *) &x=w362:refnum<file>)
        n136 = Not Equal?(x=w362, y=w361) -> (x != y?=w360:bool)
        n137 = case shown="True" w360 {
          tunnel: [w372 w375] -> w371
          tunnel: w367 -> [w372 w374]
          tunnel: w361 -> [_ w373]
          frame False {
          }
          frame True {
            n138 = Close File(refnum=w373, error in=w374) -> (error out=w375:errorcluster)  [unwired: 1 out]
          }
        }
      }
      frame "---------- UI ----------" {
        # "Template Separator\n(You can make a copy of, or modify, this frame)"
      }
      frame "UI:init" {
        # "Initialize FP objects to default values."
        n139 = Unbundle By Name(w379) -> ("objectRefsMain"=w381:T4)
        n140 = call "initFPObjectsMain.vi"("error in (no error)"=w380, "mainRefs"=w381) -> ("error out"=w378:errorcluster)  [unwired: 9 in]
      }
      frame "UI:checkConfig" {
        # "Checks for valid\nselection box choices"
        # "Checks for a single \nwavelength"
        # "Checks for\neither IL/RL"
        # "If enabled, checks for\na single used channel"
        # "Enable referencing when there is a valid channel, IL/RL selection, and wavelength chosen\nKeeps all options unlocked when in engineering mode"
        n141 = Unbundle By Name(w383) -> ("objectRefsMain.ChannelRef"=w420:refnum<vi>)
        n142 = control-ref of="Enable IL"() -> (w407:refnum<vi>)
        n143 = control-ref of="Enable RL"() -> (w417:refnum<vi>)
        n144 = control-ref of="Wavelength Enable"() -> (w416:refnum<vi>)
        n145 = Unbundle By Name(w383) -> ("objectRefsMain.StandardSelectRef"=w393:refnum<vi>)
        n146 = Unbundle By Name(w383) -> ("objectRefsMain.MethodSelectRef"=w397:refnum<vi>)
        n147 = To More Specific Class(target class=refnum<vi> refnum ("array"), reference=w420) -> (specific class reference=w419:refnum<vi>, error out=w421:errorcluster)  [unwired: 1 in]
        n148 = property class="Bool (strict)"(reference=w407) -> ("Value"=w390:bool)  [unwired: 1 in, 2 out]
        n149 = property class="Bool (strict)"(reference=w417) -> ("Value"=w412:bool)  [unwired: 1 in, 2 out]
        n150 = property class="Clust (strict)"(reference=w416) -> ("Value"=w411:T2)  [unwired: 1 in, 2 out]
        n151 = To More Specific Class(target class=refnum<vi> refnum ("Standard Selection"), reference=w393) -> (specific class reference=w392:refnum<vi>, error out=w400:errorcluster)  [unwired: 1 in]
        n152 = To More Specific Class(target class=refnum<vi> refnum ("Standard Selection"), reference=w397) -> (specific class reference=w396:refnum<vi>, error out=w398:errorcluster)  [unwired: 1 in]
        n153 = property class="Arr (strict)"(reference=w419, error in=w421) -> ("Value"=w415:bool[])  [unwired: 2 out]
        n154 = property class="Ring (strict)"(reference=w392, error in=w400) -> ("Value"=w394:u16)  [unwired: 2 out]
        n155 = property class="Ring (strict)"(reference=w396, error in=w398) -> ("Value"=w395:u16)  [unwired: 2 out]
        n156 = Boolean To (0,1)(Boolean=w415) -> (0, 1=w414:i16[])
        n157 = Cluster To Array(cluster=w411) -> (array=w408:bool[])
        n158 = Or(x=w390, y=w412) -> (x .or. y?=w391:bool)
        n159 = Add Array Elements(numeric array=w414) -> (sum=w413:i16)
        n160 = Boolean To (0,1)(Boolean=w408) -> (0, 1=w410:i16[])
        n161 = Not Equal To 0?(x=w394) -> (x != 0?=w388:bool)
        n162 = Not Equal To 0?(x=w395) -> (x != 0?=w382:bool)
        n163 = Greater Than 0?(x=w413) -> (x > 0?=w389:bool)
        n164 = Add Array Elements(numeric array=w410) -> (sum=w409:i16)
        n165 = And(x=w389, y=w388) -> (x .and. y?=w387:bool)
        n166 = Greater Than 0?(x=w409) -> (x > 0?=w402:bool)
        n167 = And(x=w387, y=w382) -> (x .and. y?=w385:bool)
        n168 = And(x=w391, y=w402) -> (x .and. y?=w384:bool)
        n169 = And(x=w385, y=w384) -> (x .and. y?=w386:bool)
        n170 = case shown="False" "Engineering Mode" {
          tunnel: w383 -> [_ w427]
          tunnel: w386 -> [_ w426]
          tunnel: w406 -> [w422 w425]
          tunnel: [w422 w424] -> w405
          tunnel: w404 -> [_ w423]
          frame True {
          }
          frame False {
            n171 = case shown="True" w426 {
              tunnel: w427 -> [_ w434]
              tunnel: w425 -> [w431 w432]
              tunnel: [w430 w432] -> w424
              tunnel: w423 -> [w429 _]
              frame False {
                n172 = call "Enqueue Message.vi"("error in (no error)"=w431, "Message"="UI:disableButton", "Message Queue"=w429) -> ("error out"=w430:errorcluster)  [unwired: 7 in, 1 out]
              }
              frame True {
                n173 = Unbundle By Name(w434) -> ("objectRefsMain.RefButtonRef"=w437:refnum<vi>)
                n174 = To More Specific Class(target class=refnum<vi> refnum ("Save Data"), reference=w437, error in=w432) -> (specific class reference=w436:refnum<vi>, error out=w438:errorcluster)
                n175 = property class="Bool"(reference=w436, error in=w438, "DisabledEnum"=T11."Enabled" ("Disabled")) -> ()  [unwired: 2 out]
              }
            }
          }
        }
      }
      frame "UI:initConfig" {
        # "Initializes all config values to their default state"
        n176 = Unbundle By Name(w442) -> ("objectRefsMain.UseSwitchRef"=w474:refnum<vi>)
        n177 = Unbundle By Name(w442) -> ("objectRefsMain.SampleIDRef"=w468:refnum<vi>)
        n178 = Unbundle By Name(w442) -> ("objectRefsMain.ChannelClusterRef"=w490:refnum<vi>)
        n179 = Unbundle By Name(w442) -> ("objectRefsMain.WavelengthRef"=w486:refnum<vi>)
        n180 = Unbundle By Name(w442) -> ("objectRefsMain.EnlableIlRef"=w485:refnum<vi>)
        n181 = Unbundle By Name(w442) -> ("objectRefsMain.EnlableRlRef"=w475:refnum<vi>)
        n182 = To More Specific Class(target class=refnum<vi> refnum ("Enable IL"), reference=w485, error in=w449) -> (specific class reference=w479:refnum<vi>, error out=w478:errorcluster)
        n183 = To More Specific Class(target class=refnum<vi> refnum ("Wavelength Enable"), reference=w486, error in=w449) -> (specific class reference=w482:refnum<vi>, error out=w481:errorcluster)
        n184 = To More Specific Class(target class=refnum<vi> refnum ("Enable IL"), reference=w475, error in=w449) -> (specific class reference=w477:refnum<vi>, error out=w476:errorcluster)
        n185 = To More Specific Class(target class=refnum<vi> refnum ("Single Channel"), reference=w474, error in=w449) -> (specific class reference=w471:refnum<vi>, error out=w472:errorcluster)
        n186 = To More Specific Class(target class=refnum<vi> refnum ("Sample Number"), reference=w468, error in=w449) -> (specific class reference=w467:refnum<vi>, error out=w469:errorcluster)
        n187 = To More Specific Class(target class=refnum<vi> refnum ("Channel Cluster"), reference=w490, error in=w449) -> (specific class reference=w488:refnum<vi>, error out=w487:errorcluster)
        n188 = property class="Clust (strict)"(reference=w488, error in=w487, "Value"=T3 {"1"=FALSE, "2"=FALSE, "3"=FALSE, "4"=FALSE, "5"=FALSE, "6"=FALSE, "7"=FALSE, "8"=FALSE, "9"=FALSE, "10"=FALSE, "11"=FALSE, "12"=FALSE, "13"=FALSE, "14"=FALSE, "15"=FALSE, "16"=FALSE, "17"=FALSE, "18"=FALSE, "19"=FALSE, "20"=FALSE, "21"=FALSE, "22"=FALSE, "23"=FALSE, "24"=FALSE}) -> ()  [unwired: 2 out]
        n189 = property class="Clust (strict)"(reference=w482, error in=w481, "Value"=T13 {"Enable 1310"=FALSE, "Enable 1490"=FALSE, "Enable 1550"=FALSE, "Enable 1625"=FALSE}) -> ()  [unwired: 2 out]
        n190 = property class="Bool (strict)"(reference=w479, error in=w478, "Value"=FALSE) -> ()  [unwired: 2 out]
        n191 = property class="Bool (strict)"(reference=w477, error in=w476, "Value"=FALSE) -> ()  [unwired: 2 out]
        n192 = property class="Bool (strict)"(reference=w471, error in=w472, "Value"=FALSE) -> ()  [unwired: 2 out]
        n193 = property class="Str"(reference=w467, error in=w469, "Value"="") -> ()  [unwired: 2 out]
        n194 = Unbundle By Name(w442) -> ("objectRefsMain.StandardSelectRef"=w460:refnum<vi>)
        n195 = Unbundle By Name(w442) -> ("objectRefsMain.MethodSelectRef"=w454:refnum<vi>)
        n196 = Unbundle By Name(w442) -> ("objectRefsMain.abortRef"=w446:refnum<vi>)
        n197 = To More Specific Class(target class=refnum<vi> refnum ("Run Time Indicator"), reference=w446) -> (specific class reference=w445:refnum<vi>, error out=w444:errorcluster)  [unwired: 1 in]
        n198 = To More Specific Class(target class=refnum<vi> refnum ("Standard Selection"), reference=w460, error in=w449) -> (specific class reference=w458:refnum<vi>, error out=w457:errorcluster)
        n199 = To More Specific Class(target class=refnum<vi> refnum ("Standard Selection"), reference=w454, error in=w449) -> (specific class reference=w453:refnum<vi>, error out=w452:errorcluster)
        n200 = control-ref of="Open Save"() -> (w440:refnum<vi>)
        n201 = call "IL-RL Standards.vi"("Input New Standard"=T1 {"Standard Name"="", "Max IL to Pass (dB)"=0.0, "Min RL to Pass (dB)"=0.0}) -> ("Standard Names"=w455:string[])  [unwired: 8 in, 1 out]
        n202 = property class="Bool"(reference=w440, "DisabledEnum"=T11."Disabled and Grayed Out" ("Disabled")) -> ()  [unwired: 1 in, 2 out]
        n203 = property class="Ring (strict)"(reference=w458, error in=w457, "Value"=u16 0, "Strings []"=w455) -> ()  [unwired: 2 out]
        n204 = property class="Ring (strict)"(reference=w453, error in=w452, "Value"=u16 0, "DisabledEnum"=T11."Disabled and Grayed Out" ("Disabled")) -> ()  [unwired: 2 out]
        n205 = property class="Bool (strict)"(reference=w445, error in=w444, "DisabledEnum"=T11."Disabled and Grayed Out" ("Disabled")) -> ()  [unwired: 2 out]
        n206 = call "Enqueue Message.vi"("error in (no error)"=w449, "Message Data"="Select Test Configurations" ("Value"), "Message"="UI:updateDisplay", "Message Queue"=w461) -> ("error out"=w464:errorcluster)  [unwired: 6 in, 1 out]
      }
      frame "UI:disableConfig" {
        # "Disables all config options\nEngineering mode disables this operation"
        n207 = Unbundle By Name(w500) -> ("objectRefsMain.EngModeRef"=w501:refnum<vi>)
        n208 = To More Specific Class(target class=refnum<vi> refnum ("Single Channel"), reference=w501, error in=w499) -> (specific class reference=w497:refnum<vi>, error out=w496:errorcluster)
        n209 = property class="Bool (strict)"(reference=w497, error in=w496) -> ("Value"=w495:bool)  [unwired: 2 out]
        n210 = case shown="False" w495 {
          tunnel: w500 -> [_ w502]
          tunnel: w499 -> [_ w503]
          frame True {
          }
          frame False {
            w511 = refnum<vi> refnum ("Enable IL")
            n211 = Unbundle By Name(w502) -> ("objectRefsMain.EnlableIlRef"=w528:refnum<vi>, "objectRefsMain.EnlableRlRef"=w510:refnum<vi>, "objectRefsMain.UseSwitchRef"=w509:refnum<vi>)
            n212 = Unbundle By Name(w502) -> ("objectRefsMain.ChannelClusterRef"=w532:refnum<vi>)
            n213 = Unbundle By Name(w502) -> ("objectRefsMain.WavelengthRef"=w529:refnum<vi>)
            n214 = Unbundle By Name(w502) -> ("objectRefsMain.StandardSelectRef"=w516:refnum<vi>)
            n215 = Unbundle By Name(w502) -> ("objectRefsMain.MethodSelectRef"=w508:refnum<vi>)
            n216 = To More Specific Class(target class=w511, reference=w528) -> (specific class reference=w524:refnum<vi>, error out=w523:errorcluster)  [unwired: 1 in]
            n217 = To More Specific Class(target class=w511, reference=w510) -> (specific class reference=w522:refnum<vi>, error out=w521:errorcluster)  [unwired: 1 in]
            n218 = To More Specific Class(target class=w511, reference=w509) -> (specific class reference=w519:refnum<vi>, error out=w520:errorcluster)  [unwired: 1 in]
            n219 = To More Specific Class(target class=refnum<vi> refnum ("Wavelength Enable"), reference=w529, error in=w503) -> (specific class reference=w527:refnum<vi>, error out=w526:errorcluster)
            n220 = To More Specific Class(target class=refnum<vi> refnum ("Standard Selection"), reference=w516, error in=w503) -> (specific class reference=w514:refnum<vi>, error out=w515:errorcluster)
            n221 = To More Specific Class(target class=refnum<vi> refnum ("Standard Selection"), reference=w508, error in=w503) -> (specific class reference=w506:refnum<vi>, error out=w507:errorcluster)
            n222 = To More Specific Class(target class=refnum<vi> refnum ("Channel Cluster"), reference=w532, error in=w503) -> (specific class reference=w531:refnum<vi>, error out=w530:errorcluster)
            n223 = property class="Clust (strict)"(reference=w531, error in=w530, "DisabledEnum"=T11."Disabled and Grayed Out" ("Disabled")) -> ()  [unwired: 2 out]
            n224 = property class="Clust (strict)"(reference=w527, error in=w526, "DisabledEnum"=T11."Disabled and Grayed Out" ("Disabled")) -> ()  [unwired: 2 out]
            n225 = property class="Bool (strict)"(reference=w524, error in=w523, "DisabledEnum"=T11."Disabled and Grayed Out" ("Disabled")) -> ()  [unwired: 2 out]
            n226 = property class="Bool (strict)"(reference=w522, error in=w521, "DisabledEnum"=T11."Disabled and Grayed Out" ("Disabled")) -> ()  [unwired: 2 out]
            n227 = property class="Bool (strict)"(reference=w519, error in=w520, "DisabledEnum"=T11."Disabled and Grayed Out" ("Disabled")) -> ()  [unwired: 2 out]
            n228 = property class="Ring (strict)"(reference=w514, error in=w515, "DisabledEnum"=T11."Disabled and Grayed Out" ("Disabled")) -> ()  [unwired: 2 out]
            n229 = property class="Ring (strict)"(reference=w506, error in=w507, "DisabledEnum"=T11."Disabled and Grayed Out" ("Disabled")) -> ()  [unwired: 2 out]
          }
        }
      }
      frame "UI:disableButton" {
        # "Disables the main buttons of the program\nEngineering mode disables this operation"
        n230 = Unbundle By Name(w539) -> ("objectRefsMain.EngModeRef"=w543:refnum<vi>)
        n231 = To More Specific Class(target class=refnum<vi> refnum ("Single Channel"), reference=w543, error in=w537) -> (specific class reference=w541:refnum<vi>, error out=w540:errorcluster)
        n232 = property class="Bool (strict)"(reference=w541, error in=w540) -> ("Value"=w538:bool)  [unwired: 2 out]
        n233 = case shown="False" w538 {
          tunnel: w539 -> [_ w575]
          tunnel: w537 -> [_ w545]
          frame True {
          }
          frame False {
            n234 = Unbundle By Name(w575) -> ("objectRefsMain.RefButtonRef"=w551:refnum<vi>, "objectRefsMain.RereferenceRef"=w550:refnum<vi>, "objectRefsMain.MeasButtonRef"=w549:refnum<vi>, "objectRefsMain.RemeasureRef"=w548:refnum<vi>, "objectRefsMain.SaveButtonRef"=w547:refnum<vi>, "objectRefsMain.SampleIDRef"=w546:refnum<vi>)
            n235 = To More Specific Class(target class=refnum<vi> refnum ("Save Data"), reference=w551, error in=w545) -> (specific class reference=w572:refnum<vi>, error out=w574:errorcluster)
            n236 = To More Specific Class(target class=refnum<vi> refnum ("Save Data"), reference=w550, error in=w545) -> (specific class reference=w567:refnum<vi>, error out=w570:errorcluster)
            n237 = To More Specific Class(target class=refnum<vi> refnum ("Save Data"), reference=w549, error in=w545) -> (specific class reference=w564:refnum<vi>, error out=w566:errorcluster)
            n238 = To More Specific Class(target class=refnum<vi> refnum ("Save Data"), reference=w548, error in=w545) -> (specific class reference=w559:refnum<vi>, error out=w562:errorcluster)
            n239 = To More Specific Class(target class=refnum<vi> refnum ("Save Data"), reference=w547, error in=w545) -> (specific class reference=w555:refnum<vi>, error out=w558:errorcluster)
            n240 = To More Specific Class(target class=refnum<vi> refnum ("Sample ID"), reference=w546, error in=w545) -> (specific class reference=w552:refnum<vi>, error out=w554:errorcluster)
            n241 = property class="Bool"(reference=w572, error in=w574, "DisabledEnum"=T11."Disabled and Grayed Out" ("Disabled")) -> ()  [unwired: 2 out]
            n242 = property class="Bool"(reference=w567, error in=w570, "DisabledEnum"=T11."Disabled and Grayed Out" ("Disabled")) -> ()  [unwired: 2 out]
            n243 = property class="Bool"(reference=w564, error in=w566, "DisabledEnum"=T11."Disabled and Grayed Out" ("Disabled")) -> ()  [unwired: 2 out]
            n244 = property class="Bool"(reference=w559, error in=w562, "DisabledEnum"=T11."Disabled and Grayed Out" ("Disabled")) -> ()  [unwired: 2 out]
            n245 = property class="Bool"(reference=w555, error in=w558, "DisabledEnum"=T11."Disabled and Grayed Out" ("Disabled")) -> ()  [unwired: 2 out]
            n246 = property class="Str"(reference=w552, error in=w554, "DisabledEnum"=T11."Disabled and Grayed Out" ("Disabled")) -> ()  [unwired: 2 out]
          }
        }
      }
      frame "UI:endRef" {
        # "Sets the buttons to ready for measure state\nEngineering mode disables this operation"
        n247 = Unbundle By Name(w581) -> ("objectRefsMain.EngModeRef"=w585:refnum<vi>)
        n248 = call "Enqueue Message.vi"("error in (no error)"=w576, "Message"="UI:endRun", "Message Queue"=w579) -> ("error out"=w578:errorcluster)  [unwired: 7 in, 1 out]
        n249 = To More Specific Class(target class=refnum<vi> refnum ("Single Channel"), reference=w585, error in=w576) -> (specific class reference=w583:refnum<vi>, error out=w582:errorcluster)
        n250 = property class="Bool (strict)"(reference=w583, error in=w582) -> ("Value"=w580:bool)  [unwired: 2 out]
        n251 = case shown="False" w580 {
          tunnel: w581 -> [_ w617]
          tunnel: w578 -> [_ w587]
          frame True {
          }
          frame False {
            n252 = Unbundle By Name(w617) -> ("objectRefsMain.RefButtonRef"=w593:refnum<vi>, "objectRefsMain.RereferenceRef"=w592:refnum<vi>, "objectRefsMain.MeasButtonRef"=w591:refnum<vi>, "objectRefsMain.RemeasureRef"=w590:refnum<vi>, "objectRefsMain.SaveButtonRef"=w589:refnum<vi>, "objectRefsMain.SampleIDRef"=w588:refnum<vi>)
            n253 = To More Specific Class(target class=refnum<vi> refnum ("Save Data"), reference=w593, error in=w587) -> (specific class reference=w614:refnum<vi>, error out=w616:errorcluster)
            n254 = To More Specific Class(target class=refnum<vi> refnum ("Save Data"), reference=w592, error in=w587) -> (specific class reference=w609:refnum<vi>, error out=w612:errorcluster)
            n255 = To More Specific Class(target class=refnum<vi> refnum ("Save Data"), reference=w591, error in=w587) -> (specific class reference=w606:refnum<vi>, error out=w608:errorcluster)
            n256 = To More Specific Class(target class=refnum<vi> refnum ("Save Data"), reference=w590, error in=w587) -> (specific class reference=w601:refnum<vi>, error out=w604:errorcluster)
            n257 = To More Specific Class(target class=refnum<vi> refnum ("Save Data"), reference=w589, error in=w587) -> (specific class reference=w597:refnum<vi>, error out=w600:errorcluster)
            n258 = To More Specific Class(target class=refnum<vi> refnum ("Sample ID"), reference=w588, error in=w587) -> (specific class reference=w594:refnum<vi>, error out=w596:errorcluster)
            n259 = property class="Bool"(reference=w614, error in=w616, "DisabledEnum"=T11."Disabled and Grayed Out" ("Disabled")) -> ()  [unwired: 2 out]
            n260 = property class="Bool"(reference=w609, error in=w612, "DisabledEnum"=T11."Enabled" ("Disabled")) -> ()  [unwired: 2 out]
            n261 = property class="Bool"(reference=w606, error in=w608, "DisabledEnum"=T11."Enabled" ("Disabled")) -> ()  [unwired: 2 out]
            n262 = property class="Bool"(reference=w601, error in=w604, "DisabledEnum"=T11."Disabled and Grayed Out" ("Disabled")) -> ()  [unwired: 2 out]
            n263 = property class="Bool"(reference=w597, error in=w600, "DisabledEnum"=T11."Disabled and Grayed Out" ("Disabled")) -> ()  [unwired: 2 out]
            n264 = property class="Str"(reference=w594, error in=w596, "DisabledEnum"=T11."Disabled and Grayed Out" ("Disabled")) -> ()  [unwired: 2 out]
          }
        }
      }
      frame "UI:endMeas" {
        # "Sets the buttons to ready for save state\nEngineering mode disables this operation"
        n265 = Unbundle By Name(w623) -> ("objectRefsMain.EngModeRef"=w627:refnum<vi>)
        n266 = call "Enqueue Message.vi"("error in (no error)"=w618, "Message"="UI:endRun", "Message Queue"=w621) -> ("error out"=w620:errorcluster)  [unwired: 7 in, 1 out]
        n267 = To More Specific Class(target class=refnum<vi> refnum ("Single Channel"), reference=w627, error in=w618) -> (specific class reference=w625:refnum<vi>, error out=w624:errorcluster)
        n268 = property class="Bool (strict)"(reference=w625, error in=w624) -> ("Value"=w622:bool)  [unwired: 2 out]
        n269 = case shown="False" w622 {
          tunnel: w623 -> [_ w659]
          tunnel: w620 -> [_ w629]
          frame True {
          }
          frame False {
            n270 = Unbundle By Name(w659) -> ("objectRefsMain.RefButtonRef"=w635:refnum<vi>, "objectRefsMain.RereferenceRef"=w634:refnum<vi>, "objectRefsMain.MeasButtonRef"=w633:refnum<vi>, "objectRefsMain.RemeasureRef"=w632:refnum<vi>, "objectRefsMain.SaveButtonRef"=w631:refnum<vi>, "objectRefsMain.SampleIDRef"=w630:refnum<vi>)
            n271 = To More Specific Class(target class=refnum<vi> refnum ("Save Data"), reference=w635, error in=w629) -> (specific class reference=w656:refnum<vi>, error out=w658:errorcluster)
            n272 = To More Specific Class(target class=refnum<vi> refnum ("Save Data"), reference=w634, error in=w629) -> (specific class reference=w651:refnum<vi>, error out=w654:errorcluster)
            n273 = To More Specific Class(target class=refnum<vi> refnum ("Save Data"), reference=w633, error in=w629) -> (specific class reference=w648:refnum<vi>, error out=w650:errorcluster)
            n274 = To More Specific Class(target class=refnum<vi> refnum ("Save Data"), reference=w632, error in=w629) -> (specific class reference=w643:refnum<vi>, error out=w646:errorcluster)
            n275 = To More Specific Class(target class=refnum<vi> refnum ("Save Data"), reference=w631, error in=w629) -> (specific class reference=w639:refnum<vi>, error out=w642:errorcluster)
            n276 = To More Specific Class(target class=refnum<vi> refnum ("Sample ID"), reference=w630, error in=w629) -> (specific class reference=w636:refnum<vi>, error out=w638:errorcluster)
            n277 = property class="Bool"(reference=w656, error in=w658, "DisabledEnum"=T11."Disabled and Grayed Out" ("Disabled")) -> ()  [unwired: 2 out]
            n278 = property class="Bool"(reference=w651, error in=w654, "DisabledEnum"=T11."Disabled and Grayed Out" ("Disabled")) -> ()  [unwired: 2 out]
            n279 = property class="Bool"(reference=w648, error in=w650, "DisabledEnum"=T11."Disabled and Grayed Out" ("Disabled")) -> ()  [unwired: 2 out]
            n280 = property class="Bool"(reference=w643, error in=w646, "DisabledEnum"=T11."Enabled" ("Disabled")) -> ()  [unwired: 2 out]
            n281 = property class="Bool"(reference=w639, error in=w642, "DisabledEnum"=T11."Enabled" ("Disabled")) -> ()  [unwired: 2 out]
            n282 = property class="Str"(reference=w636, error in=w638, "DisabledEnum"=T11."Enabled" ("Disabled")) -> ()  [unwired: 2 out]
          }
        }
      }
      frame "UI:enableConfig" {
        w668 = refnum<vi> refnum ("Enable IL")
        # "Enables all config options\nIgnores multichannel configs when no switch detected"
        n283 = Unbundle By Name(w688) -> ("Has Switch"=w667:bool)
        n284 = Unbundle By Name(w661) -> ("objectRefsMain.EnlableIlRef"=w683:refnum<vi>, "objectRefsMain.EnlableRlRef"=w675:refnum<vi>, "objectRefsMain.UseSwitchRef"=w674:refnum<vi>)
        n285 = case shown="True" w667 {
          tunnel: w674 -> [_ w692]
          tunnel: w660 -> [_ w691]
          tunnel: w661 -> [_ w690]
          tunnel: w668 -> [_ w689]
          frame False {
          }
          frame True {
            n286 = Unbundle By Name(w690) -> ("objectRefsMain.ChannelClusterRef"=w699:refnum<vi>)
            n287 = To More Specific Class(target class=w689, reference=w692) -> (specific class reference=w695:refnum<vi>, error out=w696:errorcluster)  [unwired: 1 in]
            n288 = To More Specific Class(target class=refnum<vi> refnum ("Channel Cluster"), reference=w699, error in=w691) -> (specific class reference=w698:refnum<vi>, error out=w697:errorcluster)
            n289 = property class="Bool (strict)"(reference=w695, error in=w696, "DisabledEnum"=T11."Enabled" ("Disabled")) -> ()  [unwired: 2 out]
            n290 = property class="Clust (strict)"(reference=w698, error in=w697, "DisabledEnum"=T11."Enabled" ("Disabled")) -> ()  [unwired: 2 out]
          }
        }
        n291 = Unbundle By Name(w661) -> ("objectRefsMain.StandardSelectRef"=w673:refnum<vi>)
        n292 = Unbundle By Name(w661) -> ("objectRefsMain.WavelengthRef"=w684:refnum<vi>)
        n293 = Unbundle By Name(w661) -> ("objectRefsMain.MethodSelectRef"=w666:refnum<vi>)
        n294 = To More Specific Class(target class=refnum<vi> refnum ("Standard Selection"), reference=w673, error in=w660) -> (specific class reference=w671:refnum<vi>, error out=w672:errorcluster)
        n295 = To More Specific Class(target class=refnum<vi> refnum ("Standard Selection"), reference=w666, error in=w660) -> (specific class reference=w664:refnum<vi>, error out=w665:errorcluster)
        n296 = To More Specific Class(target class=refnum<vi> refnum ("Wavelength Enable"), reference=w684, error in=w660) -> (specific class reference=w682:refnum<vi>, error out=w681:errorcluster)
        n297 = To More Specific Class(target class=w668, reference=w683) -> (specific class reference=w679:refnum<vi>, error out=w678:errorcluster)  [unwired: 1 in]
        n298 = To More Specific Class(target class=w668, reference=w675) -> (specific class reference=w677:refnum<vi>, error out=w676:errorcluster)  [unwired: 1 in]
        n299 = property class="Ring (strict)"(reference=w671, error in=w672, "DisabledEnum"=T11."Enabled" ("Disabled")) -> ()  [unwired: 2 out]
        n300 = property class="Ring (strict)"(reference=w664, error in=w665, "DisabledEnum"=T11."Enabled" ("Disabled")) -> ()  [unwired: 2 out]
        n301 = property class="Clust (strict)"(reference=w682, error in=w681, "DisabledEnum"=T11."Enabled" ("Disabled")) -> ()  [unwired: 2 out]
        n302 = property class="Bool (strict)"(reference=w679, error in=w678, "DisabledEnum"=T11."Enabled" ("Disabled")) -> ()  [unwired: 2 out]
        n303 = property class="Bool (strict)"(reference=w677, error in=w676, "DisabledEnum"=T11."Enabled" ("Disabled")) -> ()  [unwired: 2 out]
      }
      frame "UI:startRun" {
        w707 = TRUE ("Blinking")
        # "Turns the blink property for the run indicator on\nEnables abort button"
        n304 = Unbundle By Name(w702) -> ("objectRefsMain.RunTimeRef"=w712:refnum<vi>)
        n305 = Unbundle By Name(w702) -> ("objectRefsMain.abortRef"=w706:refnum<vi>)
        n306 = To More Specific Class(target class=refnum<vi> refnum ("Run Time Indicator"), reference=w712, error in=w711) -> (specific class reference=w710:refnum<vi>, error out=w709:errorcluster)
        n307 = To More Specific Class(target class=refnum<vi> refnum ("abort"), reference=w706) -> (specific class reference=w705:refnum<vi>, error out=w704:errorcluster)  [unwired: 1 in]
        n308 = property class="Bool (strict)"(reference=w710, error in=w709, "Blinking"=w707, "Label.Visible"=w707) -> ()  [unwired: 2 out]
        n309 = property class="Bool"(reference=w705, error in=w704, "DisabledEnum"=T11."Enabled" ("Disabled")) -> ()  [unwired: 2 out]
      }
      frame "UI:endRun" {
        w719 = FALSE ("Blinking")
        # "Turns the blink property for the run indicator off\nDisables abort button"
        n310 = Unbundle By Name(w714) -> ("objectRefsMain.RunTimeRef"=w724:refnum<vi>)
        n311 = Unbundle By Name(w714) -> ("objectRefsMain.abortRef"=w718:refnum<vi>)
        n312 = To More Specific Class(target class=refnum<vi> refnum ("Run Time Indicator"), reference=w724, error in=w723) -> (specific class reference=w722:refnum<vi>, error out=w721:errorcluster)
        n313 = To More Specific Class(target class=refnum<vi> refnum ("abort"), reference=w718) -> (specific class reference=w717:refnum<vi>, error out=w716:errorcluster)  [unwired: 1 in]
        n314 = property class="Bool (strict)"(reference=w722, error in=w721, "Blinking"=w719, "Label.Visible"=w719) -> ()  [unwired: 2 out]
        n315 = property class="Bool"(reference=w717, error in=w716, "DisabledEnum"=T11."Disabled and Grayed Out" ("Disabled")) -> ()  [unwired: 2 out]
      }
      frame "UI:updateDisplay" {
        # "Update the top text display with the passed string and blinks twice"
        n316 = Variant To Data(error in=w736, type="", Variant=w734) -> (data=w732:string, error out=w728:errorcluster)
        "statusMessage" <- w732
        n317 = Bundle By Name(cluster=w733, "statusMessage"=w732) -> (w731:T5)
        n318 = Unbundle By Name(w731) -> ("objectRefsMain.statusMessageRef"=w730:refnum<vi>)
        n319 = To More Specific Class(target class=refnum<vi> refnum ("Sample Number"), reference=w730, error in=w728) -> (specific class reference=w727:refnum<vi>, error out=w726:errorcluster)
        n320 = for {
          N: 2 -> [_]
          tunnel: w727 -> [w741]
          shift-right: [w738] -> _
          shift-left: w726 -> [w740]
          w737 = 100
          n321 = property class="Str"(reference=w741, error in=w740, "Text.BGColor"=u32 15830062) -> (reference out=w744:refnum<vi>, error out=w742:errorcluster)
          n322 = call "Stall Data Flow.vim"("value in"=w744, "milliseconds to wait"=w737) -> ("value out"=w743:refnum<vi>)  [unwired: 1 out]
          n323 = property class="Str"(reference=w743, error in=w742, "Text.BGColor"=u32 16777216) -> (error out=w739:errorcluster)  [unwired: 1 out]
          n324 = call "Stall Data Flow.vim"("value in"=w739, "milliseconds to wait"=w737) -> ("value out"=w738:errorcluster)  [unwired: 1 out]
        }
      }
    }
  }
  n325 = while {
    tunnel: [w753] -> w16
    tunnel: w14 -> [w757]
    tunnel: w3 -> [w755]
    tunnel: w10 -> [w747]
    tunnel: [w751] -> w11
    shift-right: [w750] -> _
    shift-left: w9 -> [w749]
    stop <- w758 stop-if-true
    # "Event Handling Loop"
    n326 = Unbundle By Name(w747) -> ("eventRegRef"=w752:refnum<event-registration>)
    n327 = Unbundle By Name(w757) -> ("SubVI"=w748:refnum<queue>, "MHL"=w756:refnum<queue>)
    n328 = event shown="[8] \"Channel Cluster.1\": Mouse Enter" {
      selector: w752 -> [_ _ _ _ _ _ _ _ _ _ _ _ _ _ _ _ _ _ _ _ _ _ w972]
      dyn-events: [_ _ _ _ _ _ _ _ _ _ _ _ _ _ _ _ _ _ _ _ _ _ w972] -> w751
      timeout: _ -> [_ _ _ _ _ _ _ _ _ _ _ _ _ _ _ _ _ _ _ _ _ _ _]
      tunnel: [_ _ _ _ _ _ _ _ _ _ _ _ _ _ _ _ _ _ _ _ TRUE ("Discard?") _ _] -> w758
      tunnel: [w761 w771 w797 w801 w805 w816 w829 w833 w845 w856 w885 w897 _ _ w918 _ _ w931 _ w961 _ _ w973] -> w754
      tunnel: w756 -> [w760 w772 w796 w800 w804 w815 w825 w837 _ w855 w884 _ _ _ _ _ _ _ _ _ _ _ w971]
      tunnel: w755 -> [_ _ _ _ _ _ _ _ _ _ _ _ _ _ _ _ _ _ _ _ _ _ _]
      tunnel: [w766 w768 w799 w803 w807 w809 w831 w838 w844 w864 w883 w907 w910 w911 w915 w922 w925 w929 w955 w958 w965 w967 w968] -> w750
      tunnel: w749 -> [w766 w768 w799 w803 w807 w809 w831 w838 w844 w864 w883 w907 w910 w911 w915 w922 w925 w929 w955 w958 w965 _ w968]
      tunnel: w748 -> [w759 w770 _ _ _ _ _ _ _ _ _ _ _ _ _ _ _ _ _ _ _ _ _]
      event "abort": Value Change {
        # "Calls the SubVIs abort command\nSets the button state to after refrerence"
        n329 = event-data() -> ()  [unwired: 1 in, 1 out]
        n330 = call "Enqueue Message.vi"("Message"="UI:endRef", "Message Queue"=w760) -> ("error out"=w763:errorcluster)  [unwired: 8 in, 1 out]
        n331 = call "Enqueue Message.vi"("Priority Message? (F)"=TRUE, "error in (no error)"=w763, "Message"="macro:abort", "Message Queue"=w759) -> ("error out"=w761:errorcluster)  [unwired: 6 in, 1 out]
      }
      event "Engineering Mode": Value Change {
        # "Executes eng mode if the entered password is correct"
        n332 = event-data() -> ("NewVal"=w767:bool)  [unwired: 1 in]
        n333 = case shown="False" w767 {
          tunnel: [TRUE w774] -> w769
          frame False {
          }
          frame True {
            n334 = call "Eng Mode Password.vi"() -> ("Password Match"=w774:bool)  [unwired: 7 in]
          }
        }
        n335 = case shown="True" w769 {
          tunnel: w772 -> [_ w788]
          tunnel: [_ w784] -> w771
          tunnel: w770 -> [_ w781]
          tunnel: w767 -> [_ w780]
          tunnel: w768 -> [w779 _]
          frame False {
            n336 = Unbundle By Name(w779) -> ("EngModeRef"=w777:refnum<vi>)
            n337 = To More Specific Class(target class=refnum<vi> refnum ("Engineering Mode"), reference=w777) -> (specific class reference=w776:refnum<vi>)  [unwired: 1 in, 1 out]
            n338 = property class="Bool (strict)"(reference=w776, "Value"=FALSE) -> ()  [unwired: 1 in, 2 out]
          }
          frame True {
            n339 = call "Enqueue Message.vi"("Message Data"=w780, "Message"="macro:engMode", "Message Queue"=w781) -> ("error out"=w782:errorcluster)  [unwired: 7 in, 1 out]
            n340 = case shown="False" w780 {
              tunnel: w788 -> [w790 w794]
              tunnel: [w789 w793] -> w787
              tunnel: [w790 w792] -> w786
              tunnel: w782 -> [w789 w791]
              frame False {
              }
              frame True {
                n341 = call "Enqueue Message.vi"("error in (no error)"=w791, "Message"="macro:engMode", "Message Queue"=w794) -> ("error out"=w793:errorcluster, "dup Message Queue"=w792:refnum<queue>)  [unwired: 7 in]
              }
            }
            n342 = call "Enqueue Message.vi"("error in (no error)"=w787, "Message"="UI:checkConfig", "Message Queue"=w786) -> ("error out"=w784:errorcluster)  [unwired: 7 in, 1 out]
          }
        }
      }
      event "Enable Switch": Value Change {
        # "Send message to MHL to allow multichannel"
        n343 = event-data() -> ()  [unwired: 1 in, 1 out]
        n344 = call "Enqueue Message.vi"("Message"="macro:channelSelect", "Message Queue"=w796) -> ("error out"=w797:errorcluster)  [unwired: 8 in, 1 out]
      }
      event "Take Reference", "Rereference": Value Change {
        # "Sends message to MHL to initialize reference procedure"
        n345 = event-data() -> ()  [unwired: 1 in, 1 out]
        n346 = call "Enqueue Message.vi"("Message"="macro:takeRef", "Message Queue"=w800) -> ("error out"=w801:errorcluster)  [unwired: 8 in, 1 out]
      }
      event "Remeasure", "Take Measurement": Value Change {
        # "Sends message to MHL to initialize measurement procedure"
        n347 = event-data() -> ()  [unwired: 1 in, 1 out]
        n348 = call "Enqueue Message.vi"("Message"="macro:takeMeas", "Message Queue"=w804) -> ("error out"=w805:errorcluster)  [unwired: 8 in, 1 out]
      }
      event "Save Data": Value Change {
        # "Sends message to MHL to initialize save procedure\nIf Sample ID is empty, send warning"
        n349 = event-data() -> ()  [unwired: 1 in, 1 out]
        n350 = Unbundle By Name(w809) -> ("SampleIDRef"=w813:refnum<vi>)
        n351 = To More Specific Class(target class=refnum<vi> refnum ("string/path"), reference=w813) -> (specific class reference=w812:refnum<vi>, error out=w814:errorcluster)  [unwired: 1 in]
        n352 = property class="Str"(reference=w812, error in=w814) -> ("Value"=w810:string)  [unwired: 2 out]
        n353 = Empty String/Path?(string/path=w810) -> (empty?=w808:bool)
        n354 = case shown="False" w808 {
          tunnel: [w817 w823] -> w816
          tunnel: w815 -> [w819 w822]
          frame True {
            n355 = call "Enqueue Message.vi"("Message Data"="Enter Sample ID" ("Message"), "Message"="UI:updateDisplay", "Message Queue"=w819) -> ("error out"=w817:errorcluster)  [unwired: 7 in, 1 out]
            n356 = One Button Dialog(message="Please add a Sample ID\nbefore saving") -> ()  [unwired: 1 in, 1 out]
          }
          frame False {
            n357 = call "Enqueue Message.vi"("Message"="macro:save", "Message Queue"=w822) -> ("error out"=w823:errorcluster)  [unwired: 8 in, 1 out]
          }
        }
      }
      event "New Test": Value Change {
        # "Sends message to MHL to new Test sequence"
        n358 = event-data() -> ()  [unwired: 1 in, 1 out]
        n359 = call "Enqueue Message.vi"("Message"="data:closeSave", "Message Queue"=w825) -> ("error out"=w827:errorcluster, "dup Message Queue"=w828:refnum<queue>)  [unwired: 8 in]
        n360 = call "Enqueue Message.vi"("error in (no error)"=w827, "Message"="macro:newTest", "Message Queue"=w828) -> ("error out"=w829:errorcluster)  [unwired: 7 in, 1 out]
      }
      event "Wavelength Enable", "Channel Cluster", "Enable RL", "IL RL Standards", "Enable IL": Value Change {
        # "Sends message to MHL to check send configs to SubVI and check config validity"
        n361 = event-data() -> ()  [unwired: 1 in, 1 out]
        n362 = call "Enqueue Message.vi"("Message"="data:sendConfig", "Message Queue"=w837) -> ("error out"=w834:errorcluster, "dup Message Queue"=w835:refnum<queue>)  [unwired: 8 in]
        n363 = call "Enqueue Message.vi"("error in (no error)"=w834, "Message"="UI:checkConfig", "Message Queue"=w835) -> ("error out"=w833:errorcluster)  [unwired: 7 in, 1 out]
      }
      event "Channel Cluster.1": Mouse Enter {
        # "Allows the channel values to be turned on and off when click dragging over the buttons"
        n364 = event-data() -> ("CtlRef"=w846:refnum<vi>)  [unwired: 1 in]
        n365 = Unbundle By Name(w844) -> ("ChannelClusterRef"=w843:refnum<vi>)
        n366 = To More Specific Class(target class=refnum<vi> refnum ("Channel Cluster"), reference=w843) -> (specific class reference=w841:refnum<vi>, error out=w840:errorcluster)  [unwired: 1 in]
        n367 = property class="Clust (strict)"(reference=w841, error in=w840) -> ("DisabledEnum"=w839:T11)  [unwired: 2 out]
        n368 = case shown="\"Enabled\"" w839 {
          tunnel: w846 -> [_ w852]
          tunnel: [_ w848] -> w845
          frame Default {
          }
          frame "Enabled" {
            n369 = property class="Bool (strict)"(reference=w852) -> (reference out=w850:refnum<vi>, error out=w849:errorcluster, "Value"=w851:bool)  [unwired: 1 in]
            n370 = Not(x=w851) -> (.not. x?=w847:bool)
            n371 = property class="Bool (strict)"(reference=w850, error in=w849, "Value"=w847) -> (error out=w848:errorcluster)  [unwired: 1 out]
          }
        }
      }
      event "Standard Selection": Value Change {
        # "Changes the values of the IL/RL Standards when the selection menu is changed\nand removes choice of dashes"
        n372 = event-data() -> ()  [unwired: 1 in, 1 out]
        n373 = call "IL-RL Standards.vi"("Input New Standard"=T1 {"Standard Name"="", "Max IL to Pass (dB)"=0.0, "Min RL to Pass (dB)"=0.0}) -> ("IL RL Standards"=w863:T17)  [unwired: 8 in, 1 out]
        n374 = case shown="1, 4" "Standard Selection" {
          selector: "Standard Selection" -> [_ _ _ _ w874]
          tunnel: w863 -> [_ _ _ _ w876]
          tunnel: [T1 {"Standard Name"="No Standard Set", "Max IL to Pass (dB)"=inf, "Min RL to Pass (dB)"=-inf} ("IL RL Standards") T1 {"Standard Name"="No Standard Set", "Max IL to Pass (dB)"=inf, "Min RL to Pass (dB)"=-inf} ("IL RL Standards") T1 {"Standard Name"="No Standard Set", "Max IL to Pass (dB)"=inf, "Min RL to Pass (dB)"=-inf} ("IL RL Standards") w871 w875] -> w862
          tunnel: [_ w866 _ _ _] -> w854
          frame 0 {
          }
          frame 1, 4 {
            n375 = control-ref of="Standard Selection"() -> (w868:refnum<vi>)
            n376 = property class="Ring (strict)"(reference=w868, "Value"=u16 0) -> (error out=w866:errorcluster)  [unwired: 1 in, 1 out]
          }
          frame 2 {
          }
          frame 3 {
            n377 = call "Custom Standard.vi"() -> ("Output Custom"=w871:T1)  [unwired: 8 in]
          }
          frame Default {
            n378 = Subtract(x=w874, y=u16 5) -> (x-y=w872:u16)
            n379 = Index Array(array=w876, index=w872) -> (element=w875:T1)
          }
        }
        "IL RL Standards" <- w862
        n380 = call "Enqueue Message.vi"("error in (no error)"=w854, "Message"="data:sendConfig", "Message Queue"=w855) -> ("error out"=w858:errorcluster, "dup Message Queue"=w859:refnum<queue>)  [unwired: 7 in]
        n381 = call "Enqueue Message.vi"("error in (no error)"=w858, "Message"="UI:checkConfig", "Message Queue"=w859) -> ("error out"=w856:errorcluster)  [unwired: 7 in, 1 out]
      }
      event "Method Selection": Value Change {
        # "Checks configs when method selection box is changed and removes choice of dashes"
        n382 = event-data() -> ()  [unwired: 1 in, 1 out]
        n383 = Unbundle By Name(w883) -> ("MethodSelectRef"=w882:refnum<vi>)
        n384 = To More Specific Class(target class=refnum<vi> refnum ("Standard Selection"), reference=w882) -> (specific class reference=w880:refnum<vi>)  [unwired: 1 in, 1 out]
        n385 = property class="Ring (strict)"(reference=w880) -> (reference out=w878:refnum<vi>, "Value"=w879:u16)  [unwired: 1 in, 1 out]
        n386 = case shown="1" w879 {
          tunnel: w878 -> [_ w892]
          tunnel: [_ w890] -> w877
          frame Default {
          }
          frame 1 {
            n387 = property class="Ring (strict)"(reference=w892, "Value"=0) -> (error out=w890:errorcluster)  [unwired: 1 in, 1 out]
          }
        }
        n388 = call "Enqueue Message.vi"("error in (no error)"=w877, "Message"="data:sendConfig", "Message Queue"=w884) -> ("error out"=w887:errorcluster, "dup Message Queue"=w888:refnum<queue>)  [unwired: 7 in]
        n389 = call "Enqueue Message.vi"("error in (no error)"=w887, "Message"="UI:checkConfig", "Message Queue"=w888) -> ("error out"=w885:errorcluster)  [unwired: 7 in, 1 out]
      }
      event "Open Save": Value Change {
        # "Opens the current save file in excel"
        n390 = event-data() -> ()  [unwired: 1 in, 1 out]
        n391 = Unbundle By Name(w907) -> ("SavePathRef"=w909:refnum<vi>)
        n392 = Automation Open(Automation Refnum="Excel._Application") -> (Automation Refnum=w905:refnum<k7>, error out=w904:errorcluster)  [unwired: 1 in, 2 out]
        n393 = property class="_Application"(reference=w905, error in=w904, "Visible"=TRUE) -> (reference out=w893:refnum<k7>, error out=w896:errorcluster, "Workbooks"=w900:refnum<k7>)
        n394 = To More Specific Class(target class=refnum<vi> refnum ("Save Path"), reference=w909) -> (specific class reference=w902:refnum<vi>)  [unwired: 1 in, 1 out]
        n395 = property class="Str"(reference=w902) -> ("Value"=w901:string)  [unwired: 1 in, 2 out]
        n396 = invoke class="Workbooks" method="Open"(reference=w900, error in=w896, "Filename"=w901) -> (error out=w898:errorcluster, "Open"=w899:refnum<k7>)  [unwired: 15 in, 16 out]
        n397 = Close Reference(reference=w899, error in (no error)=w898) -> (error out=w897:errorcluster)
        n398 = property class="_Application"(reference=w893) -> (error out=w894:errorcluster, "Hwnd"=w895:i32)  [unwired: 1 in, 1 out]
        n399 = dll-call lib="user32.dll" fn="SetForegroundWindow"(error in=w894, "Handle"=w895) -> ()  [unwired: 3 in, 3 out]
      }
      event Timeout {
        # "This case does not execute."
        # "Template Separator\n(You can make a copy of, or modify, this frame)"
        n400 = event-data() -> ()  [unwired: 1 in, 1 out]
      }
      event "menuSlider": Mouse Enter {
        w912 = TRUE  # Value
        # "Sets FP object hover state."
        n401 = event-data() -> ("CtlRef"=w913:refnum<vi>)  [unwired: 1 in]
        n402 = property class="Bool (strict)"(reference=w913, "Value"=w912) -> ()  [unwired: 1 in, 2 out]
      }
      event "menuSlider": Value Change {
        # "Sets splitter slide state."
        n403 = event-data() -> ()  [unwired: 1 in, 1 out]
        n404 = Unbundle By Name(w915) -> ("menuSplitter1Ref"=w914:refnum<vi>)
        n405 = global read "globalConstants.vi" "menuClosePosition"() -> (w921:u32)
        n406 = global read "globalConstants.vi" "menuOpenPosition"() -> (w920:u32)
        n407 = To More Specific Class(target class=refnum<vi> refnum ("Splitter Refnum"), reference=w914) -> (specific class reference=w916:refnum<vi>, error out=w919:errorcluster)  [unwired: 1 in]
        n408 = call "MenuSlider.vi"("Error In"=w919, "Open Position"=w920, "Close Position"=w921, "Splitter Refnum"=w916) -> ("Error Out"=w918:errorcluster)  [unwired: 7 in]
      }
      event "menuSlider": Mouse Leave {
        # "Sets FP object hover state."
        n409 = event-data() -> ("CtlRef"=w924:refnum<vi>)  [unwired: 1 in]
        n410 = property class="Bool (strict)"(reference=w924, "Value"=FALSE) -> ()  [unwired: 1 in, 2 out]
      }
      event "moduleSlider": Mouse Enter {
        # "Sets FP object hover state."
        n411 = event-data() -> ("CtlRef"=w927:refnum<vi>)  [unwired: 1 in]
        n412 = property class="Bool (strict)"(reference=w927, "Value"=TRUE) -> ()  [unwired: 1 in, 2 out]
      }
      event "moduleSlider": Value Change {
        w930 = refnum<vi> refnum ("Splitter Refnum")
        # "Sets splitter slide state."
        n413 = event-data() -> ()  [unwired: 1 in, 1 out]
        n414 = global read "globalConstants.vi" "menuOpenPosition"() -> (w938:u32)
        n415 = Unbundle By Name(w929) -> ("moduleSplitter1Ref"=w935:refnum<vi>, "menuSplitter1Ref"=w928:refnum<vi>)
        n416 = To More Specific Class(target class=w930, reference=w928) -> (specific class reference=w934:refnum<vi>, error out=w933:errorcluster)  [unwired: 1 in]
        n417 = property on="Property Node" class="Splitter"(reference=w934, error in=w933) -> (error out=w932:errorcluster, "Position"=w937:i32)  [unwired: 1 out]
        n418 = Equal?(x=w937, y=w938) -> (x = y?=w936:bool)
        n419 = case shown="False" w936 {
          tunnel: w935 -> [w939 w947]
          tunnel: w932 -> [w942 w951]
          tunnel: [w943 w950] -> w931
          tunnel: w930 -> [w941 w949]
          frame True {
            w944 = enum16{"Reset", "Slide"}."Reset"  # State
            n420 = To More Specific Class(target class=w941, reference=w939) -> (specific class reference=w940:refnum<vi>)  [unwired: 1 in, 1 out]
            n421 = global read "globalConstants.vi" "moduleClosePosition2"() -> (w946:u32)
            n422 = global read "globalConstants.vi" "moduleOpenPosition2"() -> (w945:u32)
            n423 = call "MenuSlider.vi"("State"=w944, "Error In"=w942, "Open Position"=w945, "Close Position"=w946, "Splitter Refnum"=w940) -> ("Error Out"=w943:errorcluster)  [unwired: 6 in]
          }
          frame False {
            w952 = enum16{"Reset", "Slide"}."Reset"  # State
            n424 = To More Specific Class(target class=w949, reference=w947) -> (specific class reference=w948:refnum<vi>)  [unwired: 1 in, 1 out]
            n425 = global read "globalConstants.vi" "moduleClosePosition"() -> (w954:u32)
            n426 = global read "globalConstants.vi" "moduleOpenPosition"() -> (w953:u32)
            n427 = call "MenuSlider.vi"("State"=w952, "Error In"=w951, "Open Position"=w953, "Close Position"=w954, "Splitter Refnum"=w948) -> ("Error Out"=w950:errorcluster)  [unwired: 6 in]
          }
        }
      }
      event "moduleSlider": Mouse Leave {
        # "Sets FP object hover state."
        n428 = event-data() -> ("CtlRef"=w957:refnum<vi>)  [unwired: 1 in]
        n429 = property class="Bool (strict)"(reference=w957, "Value"=FALSE) -> ()  [unwired: 1 in, 2 out]
      }
      event Panel Resize; Pane Size {
        w964 = T18 {"Left"=6, "Top"=0}  # Position
        # "Resets position of FP objects during resize."
        n430 = event-data() -> ()  [unwired: 1 in, 1 out]
        n431 = Unbundle By Name(w958) -> ("menuSliderRef"=w963:refnum<vi>, "moduleSliderRef"=w962:refnum<vi>)
        n432 = property on="Property Node" class="GObj"(reference=w963, "Position"=w964) -> (error out=w960:errorcluster)  [unwired: 1 in, 1 out]
        n433 = property on="Property Node" class="GObj"(reference=w962, "Position"=w964) -> (error out=w959:errorcluster)  [unwired: 1 in, 1 out]
        n434 = Merge Errors(w960, w959) -> (w961:errorcluster)
      }
      event User Event {
        # "Exit EHL."
        n435 = event-data() -> ()  [unwired: 1 in, 1 out]
      }
      event User Event {
        # "Send objectRefsMain to EHL."
        n436 = event-data() -> ("objectRefsMain"=w967:T4)  [unwired: 1 in]
      }
      event Panel Close? {
        w970 = TRUE  # Discard?
        # "Send message to MHL to execute macro:initExit procedure."
        n437 = event-data() -> ()  [unwired: 1 in, 1 out]
        n438 = call "Enqueue Message.vi"("Message"="macro:initExit", "Message Queue"=w971) -> ("error out"=w973:errorcluster)  [unwired: 8 in, 1 out]
        n439 = event-data("Discard?"=w970) -> ()  [unwired: 1 in, 1 out]
      }
    }
    n440 = call <vilib>:"Simple Error Handler.vi"("error in (no error)"=w754) -> ("error out"=w753:errorcluster)  [unwired: 4 in, 4 out]
  }
  n441 = Unbundle By Name(w3) -> ("SubViRef"=w7:refnum<vi>)
  n442 = invoke on="SubVI Subpanel" class="SubPnl" method="Insert VI"(error in=w8, "VI Ref"=w7) -> (error out=w2:errorcluster)  [unwired: 2 in, 3 out]
  n443 = Unbundle(w2) -> ("code"=w1:i32)  [unwired: 2 out]
  n444 = case shown="1144" w1 {
    frame 0, Default {
    }
    frame 1144 {
      n445 = One Button Dialog(message="Device program already in\nuse. Close all and restart") -> ()  [unwired: 1 in, 1 out]
    }
  }
  n446 = Unregister For Events(event registration refnum=w11, error in=w16) -> (error out=w18:errorcluster)
  n447 = Merge Errors(w18, w15, w2) -> (w19:errorcluster)
  n448 = call "Destroy User Event - Stop.vi"("error in (no error)"=w19) -> ("error out"=w17:errorcluster)  [unwired: 10 in]
  n449 = disable-structure shown="RUN_TIME_ENGINE==True" {
    disable-tunnel: w17 -> [_ _]
    frame condition #0 (active) {
    }
    frame condition #1 {
      # "Call Quit LabVIEW if running as a built application."
      n450 = Quit LabVIEW() -> ()  [unwired: 1 in]
    }
  }
